vi "Text control 2 v6.7.vi"() -> ()   [LabVIEW 2016]
panel:
  in  "Tab Control":enum32{"Main", "Other parameters"}(tab)
  in  "Plot sample extrema vs time":bool
  out "Line running":i32
  out "Total lines":i32
  out "Path":path=path "C:/users/rlp38/09Apr2009LTtesting/test2.txt"
  out "I vs Vg":cluster{"Y data in":dbl[], "X data in":dbl[]}[](graph)
  out "Is max":dbl format="%.2e"
  out "Id max":dbl format="%.2e"
  out "Ig max":dbl format="%.2e"
  out "Imax vs time":cluster{"Y data in":dbl[], "X data in":dbl[]}[](graph)
  out "Imin vs time":cluster{"Y data in":dbl[], "X data in":dbl[]}[](graph)
  out "I vs Vd":cluster{"Y data in":dbl[], "X data in":dbl[]}[](graph)
  in  "Script":string="#pulsedstressV d 0.03 20 0 0.5 0.0827 5\n#\n#itime m\n#gaterangemode a\n#drainrangemode a\n#pulsed on 0.05 0 0.02\n#transfer d -10 40 1 5 40 35\n#transfer d -10 40 1 5 40 35\n#transfer d -10 40 1 5 40 35\n#output d 0 40 20 0 40 1\n#\n#\n#sample 1 0.008 221 6 0.003\n#samplei 400e-6 200 6 0.002 0.1\n#vsu2pulse -10 4\n#\n#stressV 0.016 0.03 2e-4 0.1e-3 11\n#stressI 220e-7 0.08 15\n#transfer s -1 1 0.5 -0.005 0.005 0.005\n#output s 0 0 0 -0.008 0.008 0.002"
  out "Command running:":string
  out "Serial port data":string
  out "Elapsed Time":dbl caption="Elapsed Time (s)"
  in  "Time Units":u16(ring)=1 items=["Seconds", "Minutes", "Hours"]
  in  "Time Offset":dbl caption="Set Start Time (s)"
  in  "Reset":bool
  in  "Auto Reset":bool
  in  "integration time":u32(slide) max=2 step=1 scale=0.0..2.0
  out "Is on":dbl format="%.2e"
  out "Id on":dbl format="%.2e"
  out "Ig on":dbl format="%.2e"
  out "Ion vs time":cluster{"Y data in":dbl[], "X data in":dbl[]}[](graph)
  out "Ioff vs time":cluster{"Y data in":dbl[], "X data in":dbl[]}[](graph)
  out "Ig min":dbl format="%.2e"
  out "Id min":dbl format="%.2e"
  out "Is min":dbl format="%.2e"
  out "Is off":dbl format="%.2e"
  out "Id off":dbl format="%.2e"
  out "Ig off":dbl format="%.2e"
  in  "Integration time (long)":dbl=0.32 min=0.04 max=2.0 step=0.02 format="%.2f"
  in  "Integration time (short)":dbl=0.0019 min=8e-05 max=0.0019 step=8e-05 format="%^.0e"
  in  "Drain: Compliance":dbl=0.001 format="%.8f"
  in  "Gate: Compliance":dbl=0.001 format="%.8f"
  in  "Interrupt scan":bool
  in  "Interrupt program":bool
  in  "Plot output curve extrema vs time":bool
  in  "Plot transfer curve extrema vs time":bool
  out "I vs time (Bias Stress)":cluster{"Y data in":dbl[], "X data in":dbl[]}[](graph)
  in  "Gate Range\nmode":u16(ring) items=["Auto", "Limited", "Fixed"]
  in  "Gate Range":u8(slide)=6 max=11 scale=0.0..11.0
  in  "Source/Drain\nRange mode":u16(ring) items=["Auto", "Limited", "Fixed"]
  in  "Source/Drain Range":u8(slide)=6 max=11 scale=0.0..11.0
  in  "Panel Controls":T1={"Emergency Stop"=refnum, "TransGraph Max"=1e-05, "Text/Graph (text=false)"=TRUE} {"TransGraph Max" format="%.2e"}
  in  "Panel Controls 2":T2={"Emergency Stop"=refnum, "TransGraph Max"=1e-05, "Text/Graph (text=false)"=TRUE, "TransGraph Min"=1e-11} {"TransGraph Min" format="%.2e"; "TransGraph Max" format="%.2e"}
  out "error out":errorcluster
  in  "Delay before read (ms)":u32=1000
  in  "byte count":u32=64
  in  "Serial End Mode for Reads":u16(ring)=2 items=["None", "LastBit", "TermChar"]
  in  "Timeout (ms)":u32=10000
  in  "Enable Termination\nChar (T)":bool=TRUE
  in  "Termination char\n(0xA = '\\n' = LF)\n(0xD = '\\r' = CR)":u8=13 format="%.0x"
  in  "flow control":u16(ring) items=["None"=0, "XON/XOFF"=1, "RTS/CTS"=2, "DTR/DSR"=4]
  in  "stop bits":u16(ring)=10 items=["1.0"=10, "1.5"=15, "2.0"=20]
  in  "parity":u16(ring) items=["None", "Odd", "Even", "Mark", "Space"]
  in  "data bits":u16=8 min=5 max=8 step=1
  in  "VISA resource name":refnum<visa-resource-name>="COM6"
  in  "baud rate":u32=9600
  out "Timings Indicator":T3
  in  "Timings (overwritten by the Front Panel)":T4={"integration time"=0, "Short/Long integration time"=0.00064, "hold time (sec)"=0.0, "delay time (sec)"=0.0, "Step Time (0 disables)"=0.0, "sweep method"=0, "Pulse period"=0.005, "Base voltage"=0.0, "Pulse width"=0.0005} {"Pulse width" min=0.0005 max=0.1 step=0.0001 format="%.4f"; "Base voltage" format="%^.4e"; "Pulse period" min=0.005 max=1.0 step=0.0001 format="%.4f"; "sweep method" items=["Continuous", "Pulsed"]; "Step Time (0 disables)" format="%.2f"; "delay time (sec)" format="%.4f"; "hold time (sec)" format="%.4f"; "Short/Long integration time" format="%^.0e"; "integration time" scale=0.0..2.0}
  in  "SMU4":cluster{"on/off":bool, "Voltage":dbl} {"Voltage" min=-100.0 max=100.0 format="%.2f"}
  in  "Full Reset":bool
  in  "Standby":T5
  out "SMU4 Indicator":cluster{"on/off":bool, "Voltage":dbl} {"Voltage" min=-100.0 max=100.0 format="%.2f"}
  in  "Gate":T6={"Gate Start"=0.0, "Gate Stop"=2.0, "Gate Step (linear only)"=1.0, "Gate Compliance"=0.0001, "Gate PComp"=0.0, "Range mode"=0, "Range"=6} {"Range" max=11 scale=0.0..11.0; "Range mode" items=["Auto", "Limited", "Fixed"]; "Gate PComp" format="%^.2e"; "Gate Compliance" format="%^.2e"; "Gate Step (linear only)" format="%^.4e"; "Gate Stop" format="%^.4e"; "Gate Start" format="%^.4e"}
  in  "Drain 2":T7={"Drain Start"=0.0, "Drain Stop"=2.0, "Drain Compliance"=0.0001, "Drain Step"=1.0, "Drain PComp"=0.0, "Range mode"=0, "Range"=6} {"Range" max=11 scale=0.0..11.0; "Range mode" items=["Auto", "Limited", "Fixed"]; "Drain PComp" format="%^.2e"; "Drain Step" format="%^.4e"; "Drain Compliance" format="%^.2e"; "Drain Stop" format="%^.4e"; "Drain Start" format="%^.4e"}
  # "Time"
  # "Syntax:\nitime [s|m|l] time(sec): [s|m|l] determines the integration time setting (small|medium|long) and time sets the value.\nNOTE: The value of the integration time has to be within the range allowed by its category (s|m|l), otherwise, the closest value will be used. (e.g. if the category is set to short but the time value is very long, the actual value used will be the maximum short integration time.\nIntegration times:\n    Short: Default: 640 us. Range: 8E-5 - 1.92E-3 seconds.\n    Medium: Fixed at 1 NPL cycle (0.02 seconds).\n    Long: Default: 16 NPL cycles (0.32 seconds). Range: 2-100 NPL cycles (0.04 seconds - 2 seconds).\ngaterangemode [a|l|f]\ndrainrangemode [a|l|f]\npulsed [on|off] PulsePeriod(sec) PulseBaseVoltage PulseONWidth(sec)\nstandby [on l off]\nwait NumMilliseconds\nwait-min NumMinutes\n# texthere = comment\nSMU4 [ON|OFF] Voltage\ntransfer [s|d] VgStart VgStop VgStep VdStart VdStop VdStep\noutput [s|d] VgStart VgStop VgStep VdStart VdStop VdStep\nsample Vg Vd NumSamples Time(s) SampleInterval(s)\nsamplei Idg NumSamples Time(s) SampleInterval(s) VDGcompliance\n100 samples is approximately 13 seconds with medium integration\n# if in doubt use SampleInterval(s) = 0.004\n    NOTE: When doing bias stress measurements, set the Time Units to \"Seconds\", as the \"sample\" command has been configured to give the output to seconds.\nstressV VG VD IGcompliance IDcompliance Duration(sec)\nstressI IDG VDGcompliance Duration(sec)\nvsu2pulse Bias Duration(s)\npulsedstressV [s|d] VEstop VgON VgOFF Period(s) PulseONwidth(s) Vd\nsample-fpp Vg Vd NumSamples Time\nresample-fpp Vg Vd\ntransfer-fpp [s|d] VgStart VgStop VgStep VdStart VdStop VdStep\noutput-fpp [s|d] VgStart VgStop VgStep VdStart VdStop VdStep\nserial SerialPortCommand"
  # "1\n2\n3\n4\n5\n6\n7\n8\n9\n10\n11\n12\n13\n14\n15\n16\n17\n18\n19\n20"
  # "Serial port settings"
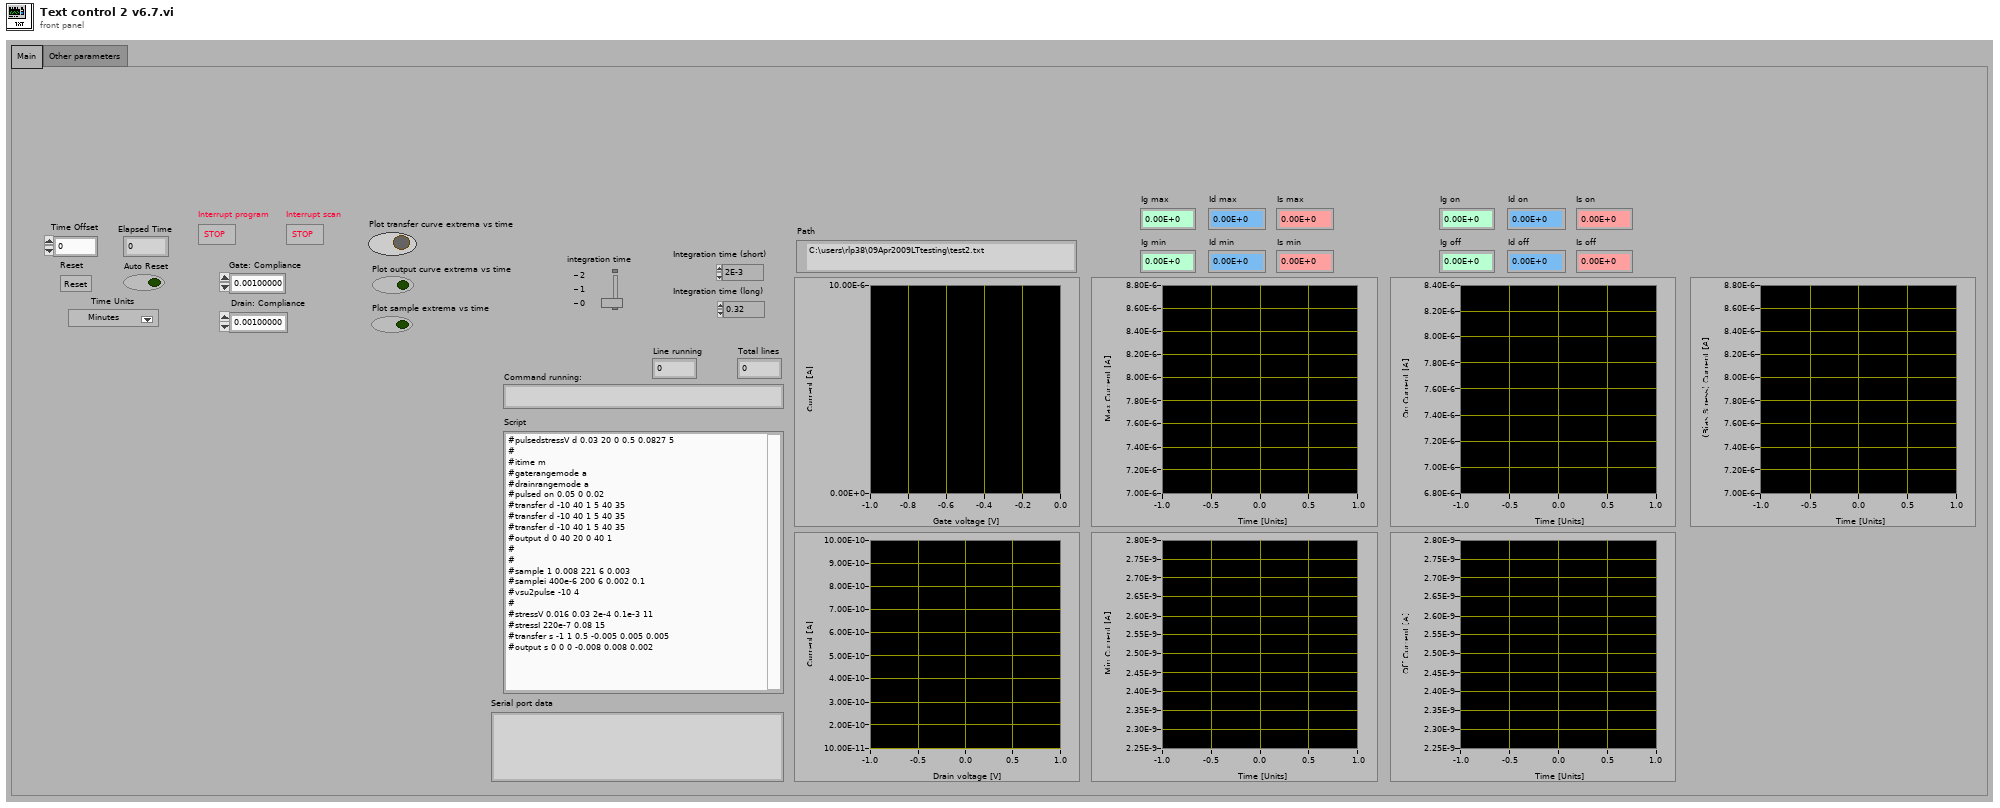
[diagram p1: front panel]
types:
  T1 = cluster{"Emergency Stop":refnum<vi>, "TransGraph Max":dbl, "Text/Graph (text=false)":bool}
  T2 = cluster{"Emergency Stop":refnum<vi>, "TransGraph Max":dbl, "Text/Graph (text=false)":bool, "TransGraph Min":dbl}
  T3 = cluster{"integration time (0:s, 1:m, 2:l)":u32, "Short/Long integration time":dbl, "hold time (sec)":dbl, "delay time (sec)":dbl, "Step Time (0 disables)":dbl, "sweep method":u16, "Pulse period":dbl, "Base voltage":dbl, "Pulse width":dbl}
  T4 = cluster{"integration time":u32, "Short/Long integration time":dbl, "hold time (sec)":dbl, "delay time (sec)":dbl, "Step Time (0 disables)":dbl, "sweep method":u16, "Pulse period":dbl, "Base voltage":dbl, "Pulse width":dbl}
  T5 = cluster{"Gate Standby":bool, "Drain Standby":bool}
  T6 = cluster{"Gate Start":dbl, "Gate Stop":dbl, "Gate Step (linear only)":dbl, "Gate Compliance":dbl, "Gate PComp":dbl, "Range mode":u16, "Range":u8}
  T7 = cluster{"Drain Start":dbl, "Drain Stop":dbl, "Drain Compliance":dbl, "Drain Step":dbl, "Drain PComp":dbl, "Range mode":u16, "Range":u8}
  T8 = enum16{"open", "replace", "create", "open or create", "replace or create", "replace or create with confirmation"}
  T9 = cluster{"V2 Start":dbl, "V2 Step":dbl, "Number of points":i32}
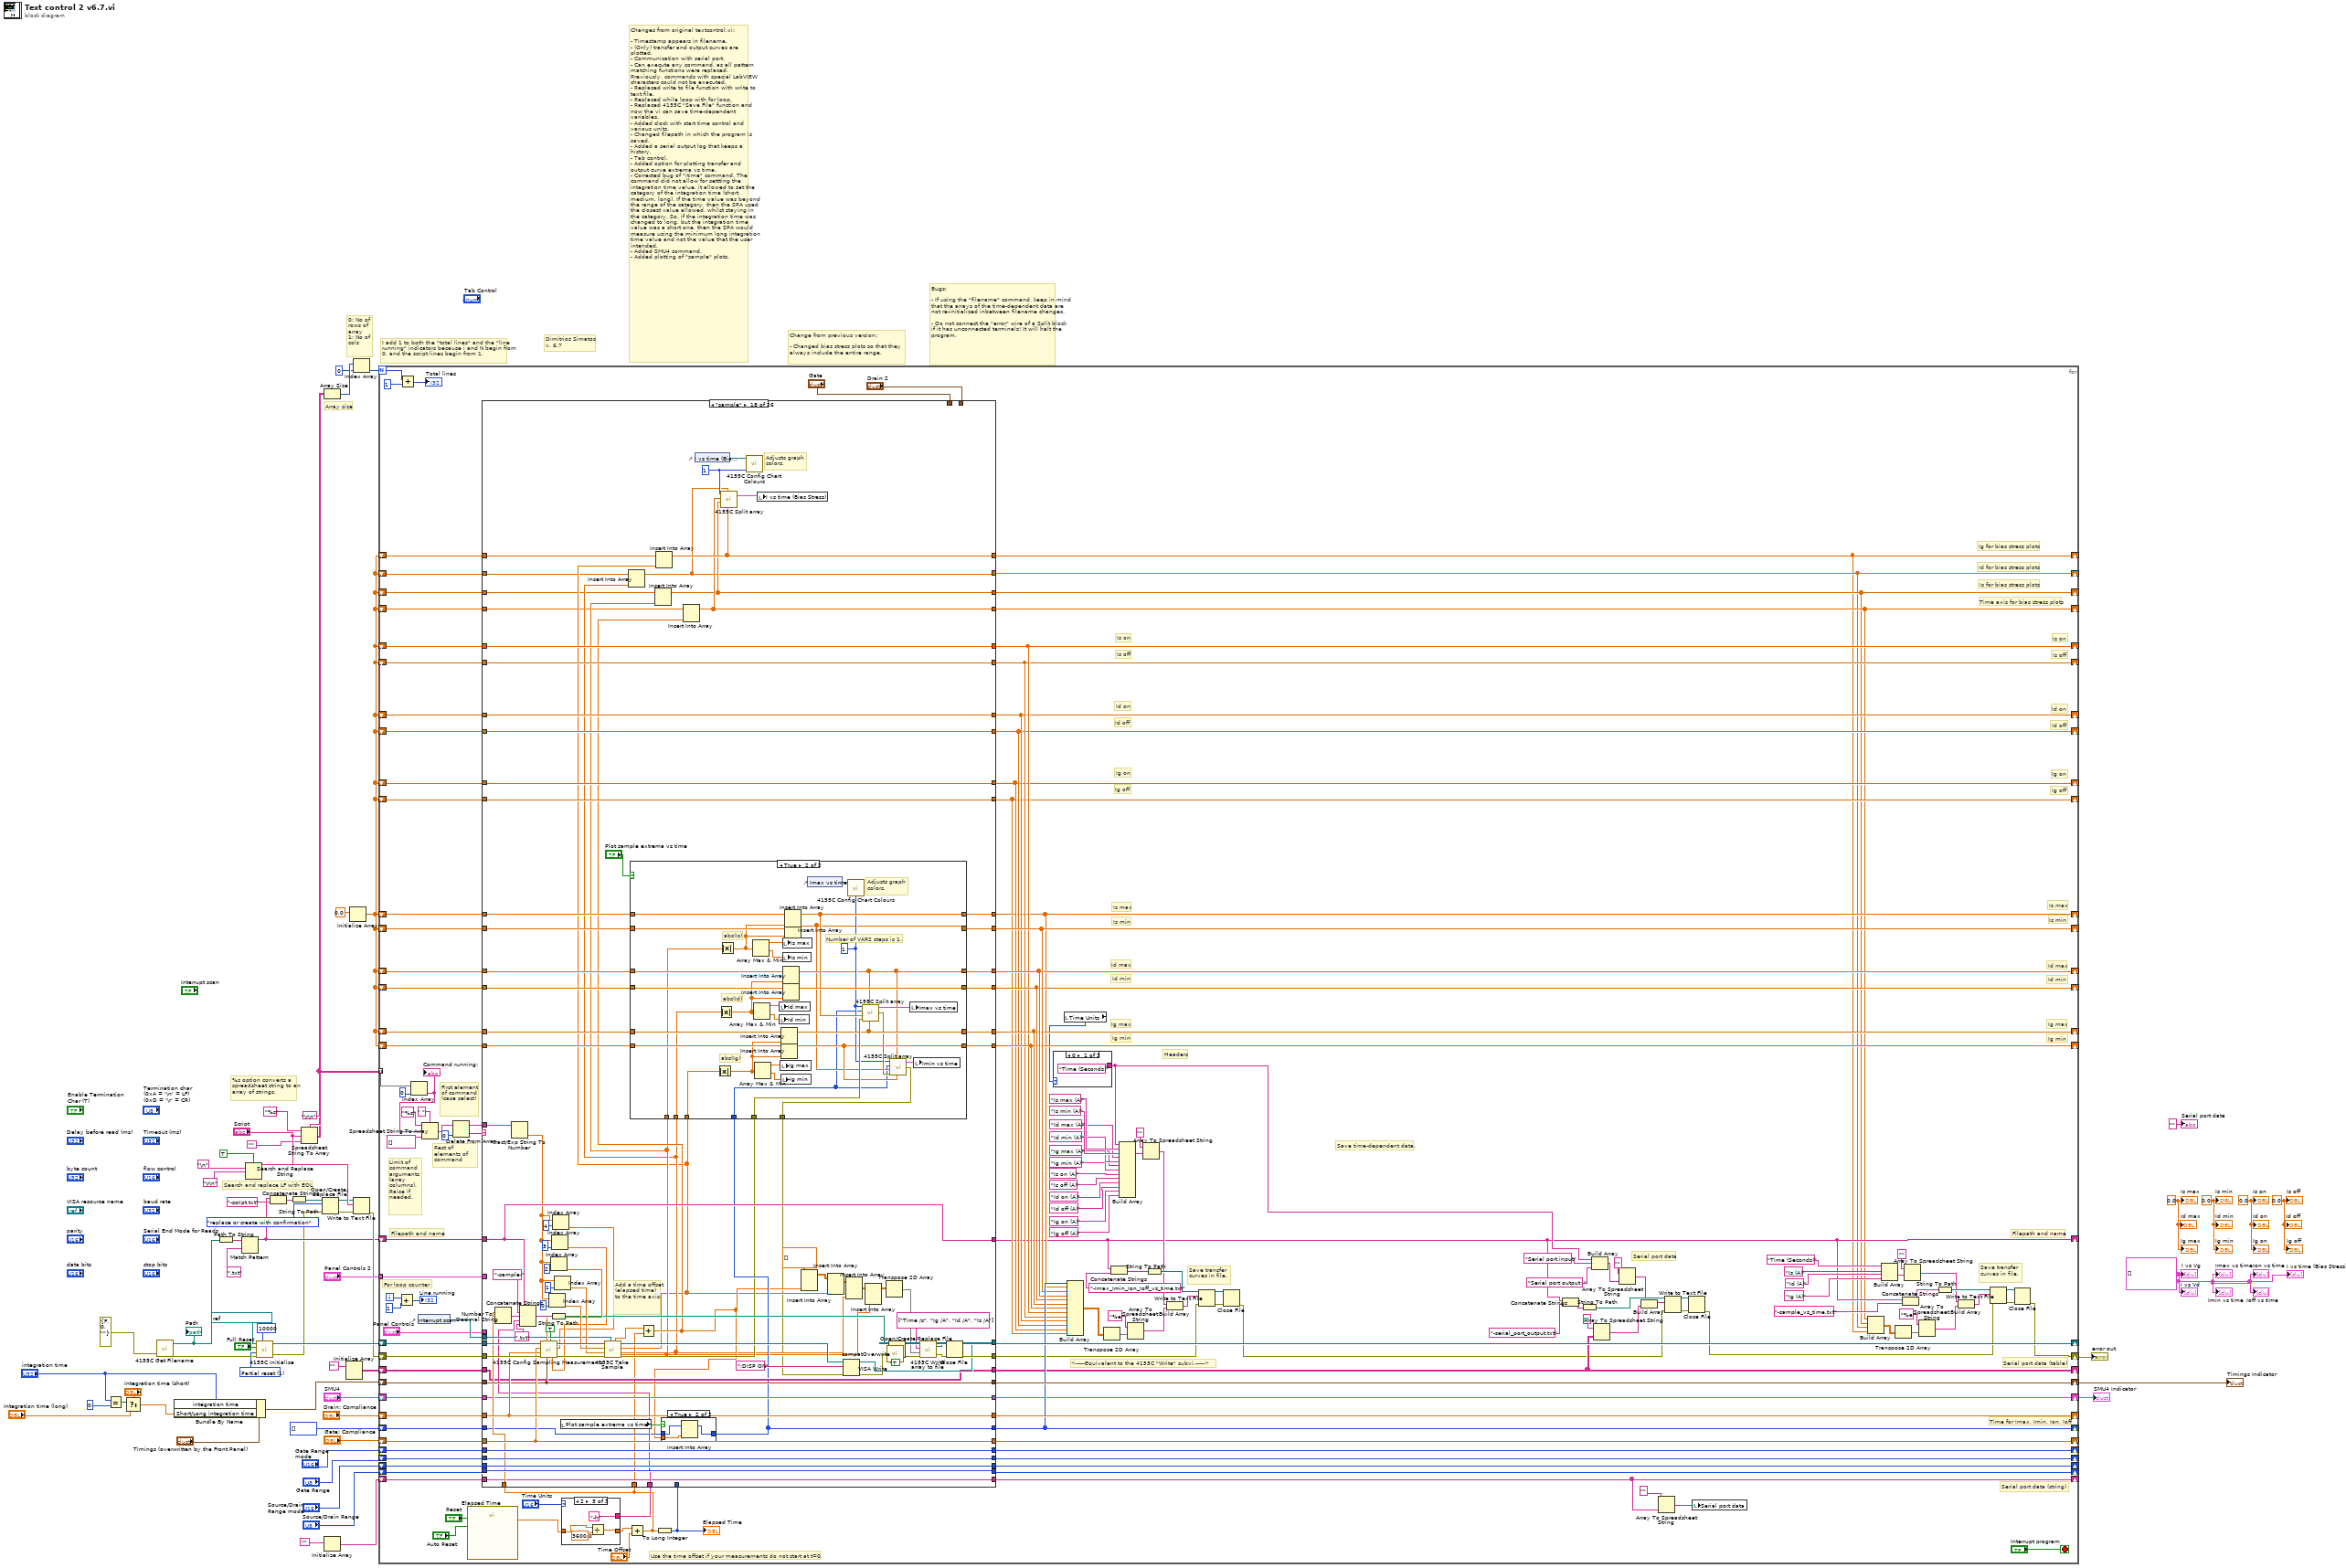
[diagram p0: block diagram]
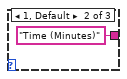
[diagram p2: hidden frame]
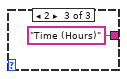
[diagram p3: hidden frame]
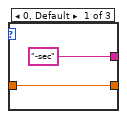
[diagram p4: hidden frame]
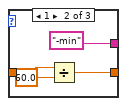
[diagram p5: hidden frame]
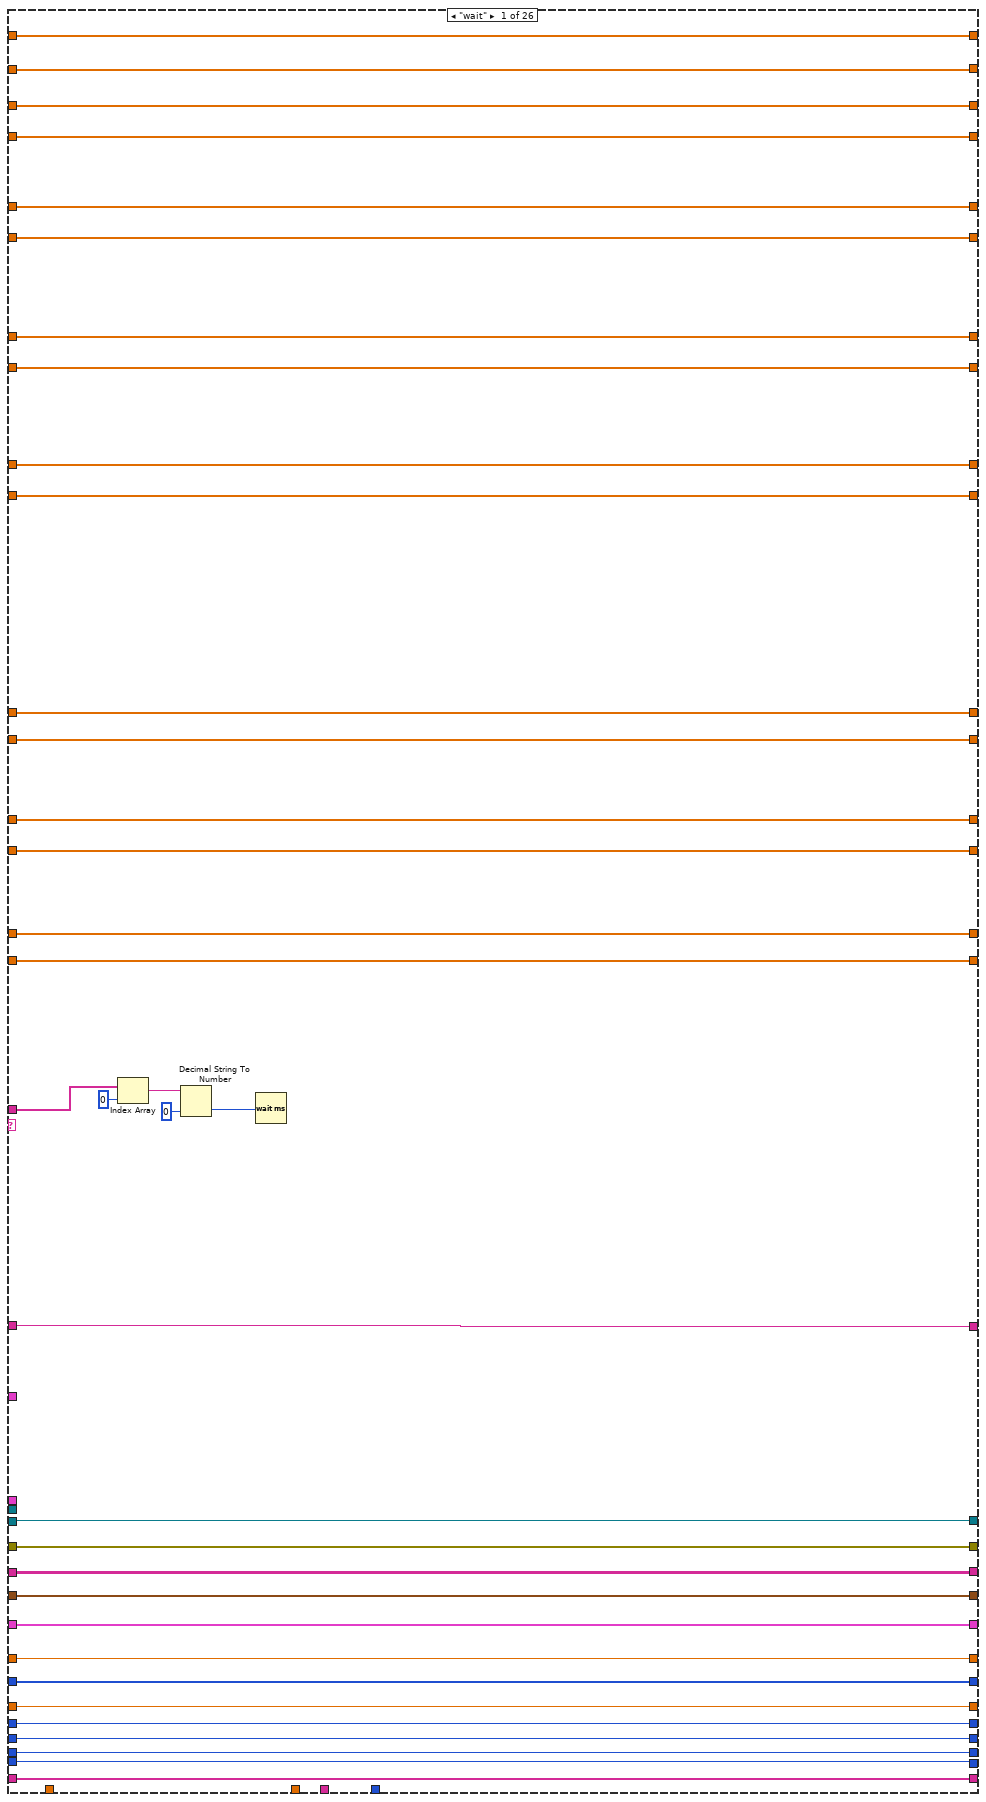
[diagram p6: hidden frame]
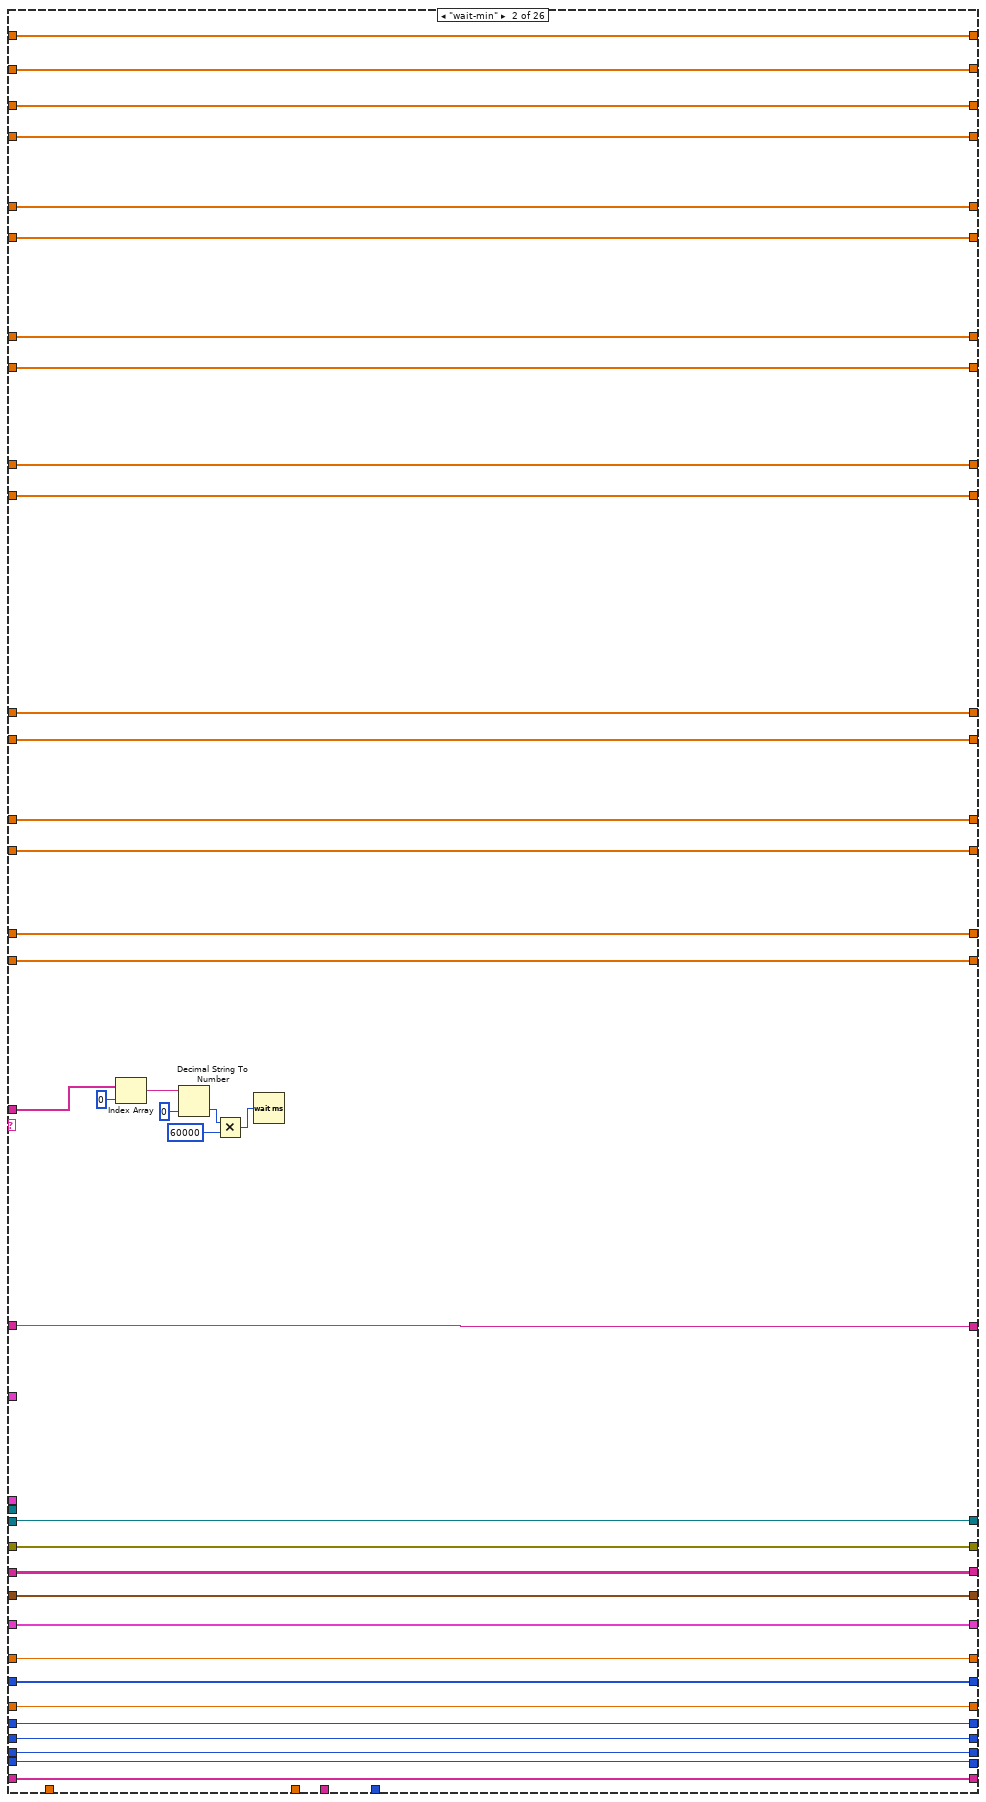
[diagram p7: hidden frame]
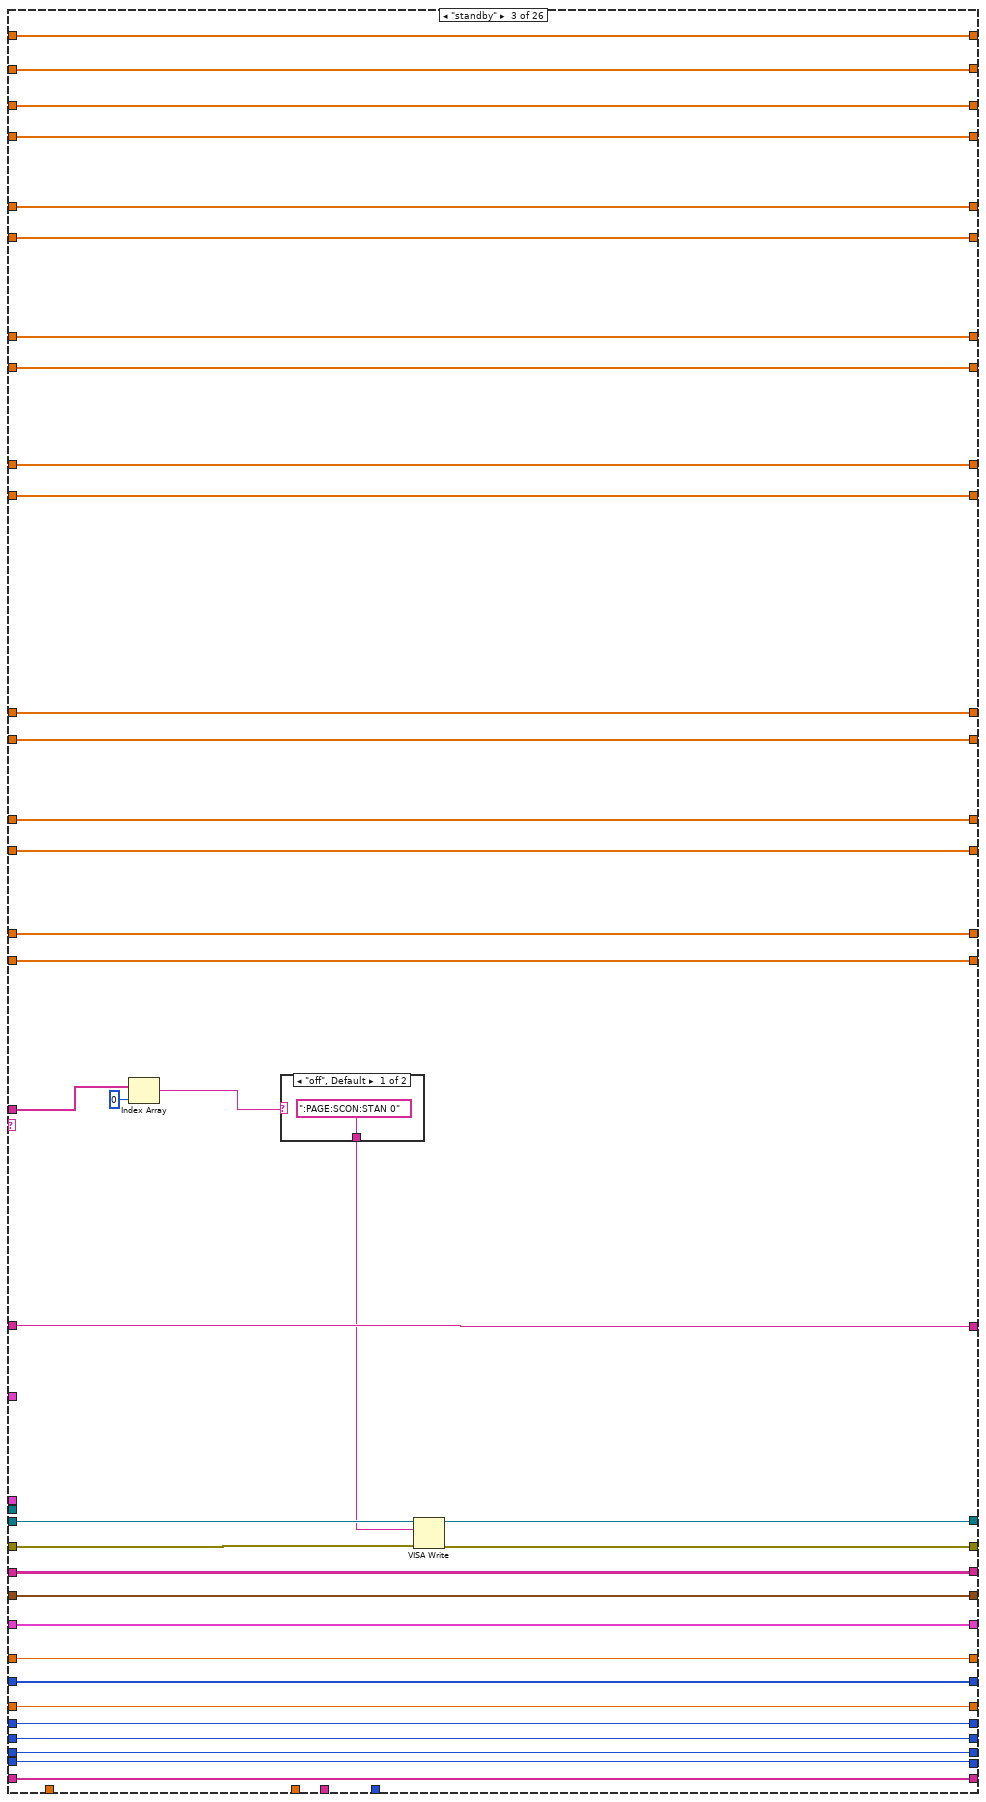
[diagram p8: hidden frame]
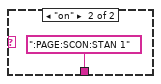
[diagram p9: hidden frame]
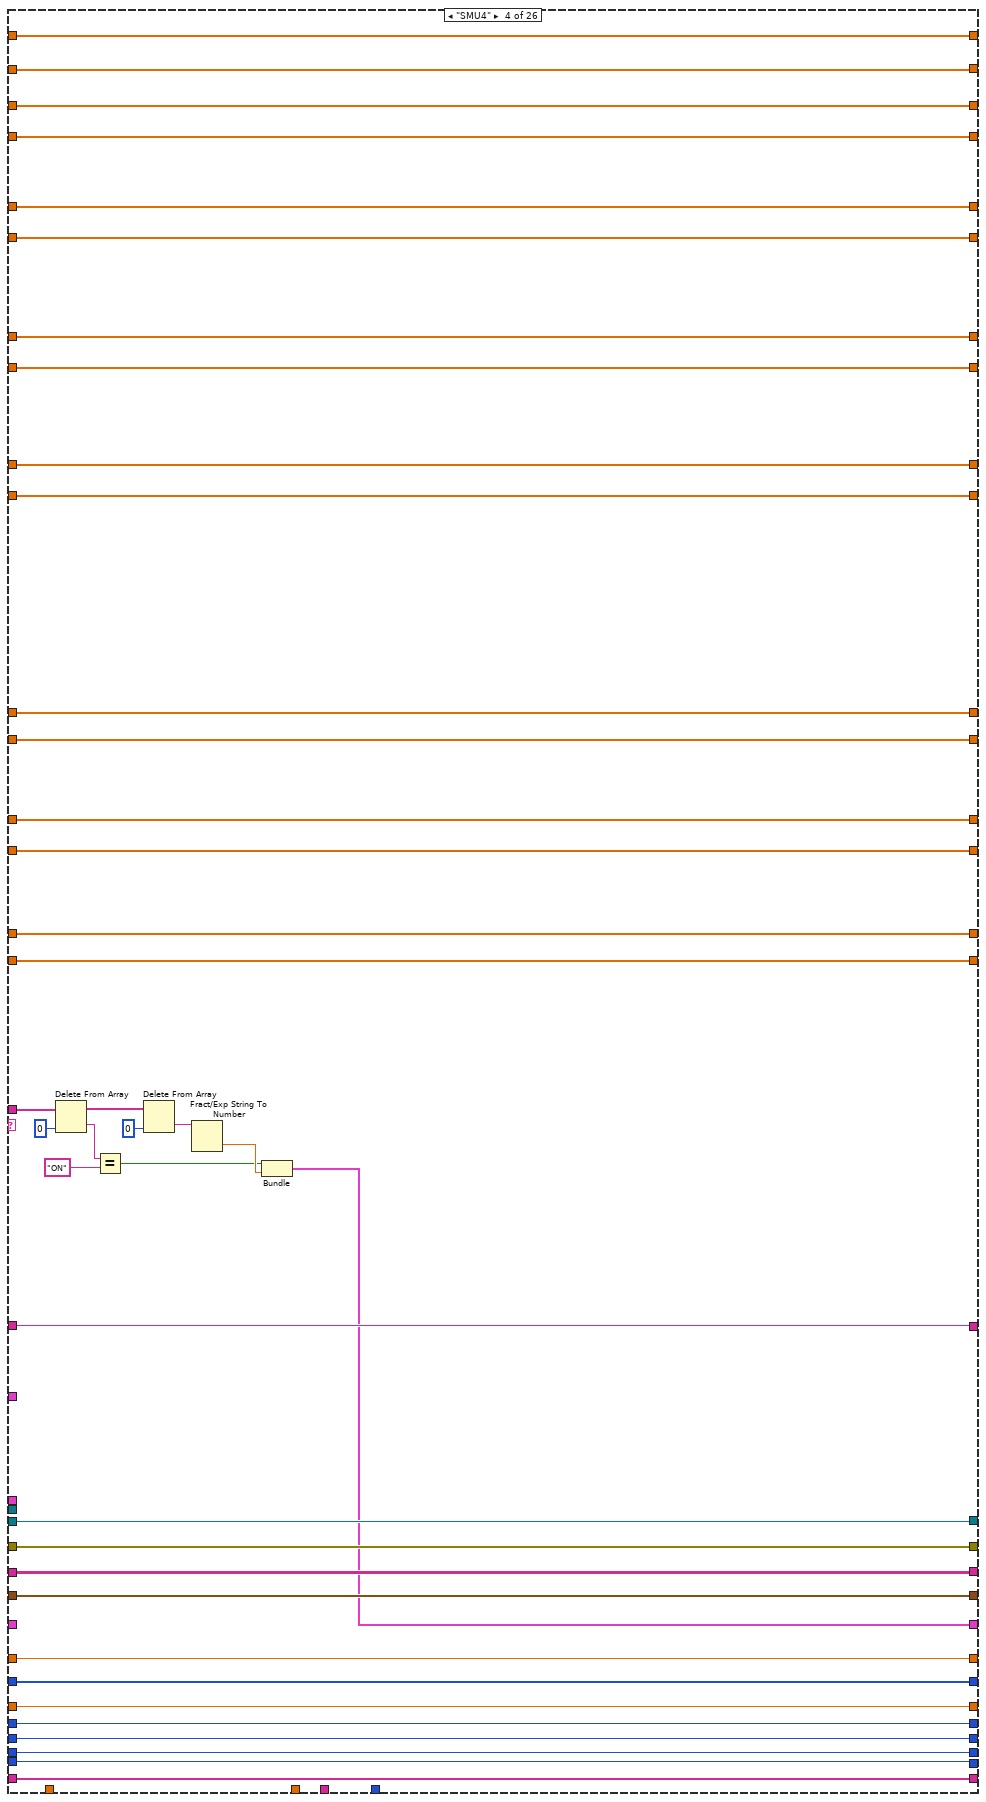
[diagram p10: hidden frame]
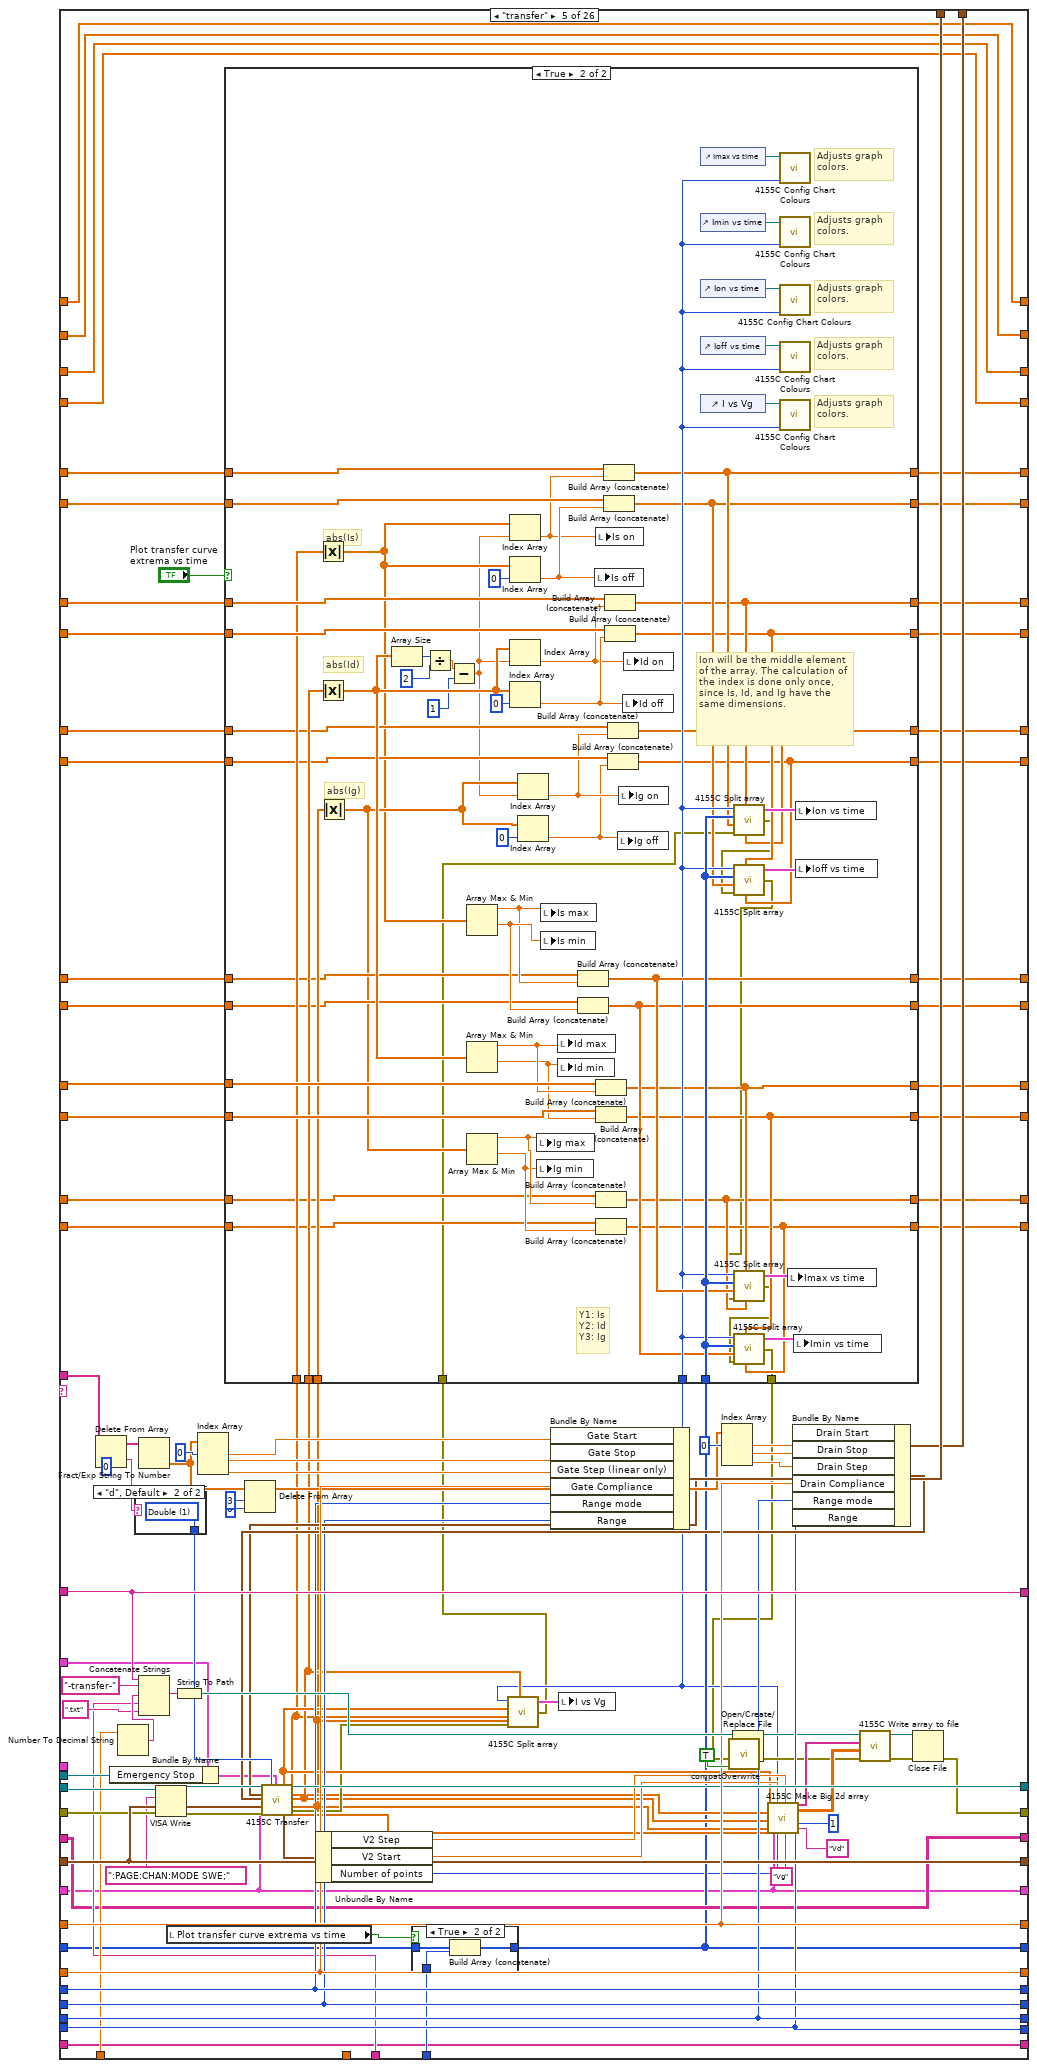
[diagram p11: hidden frame]
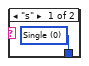
[diagram p14: hidden frame]
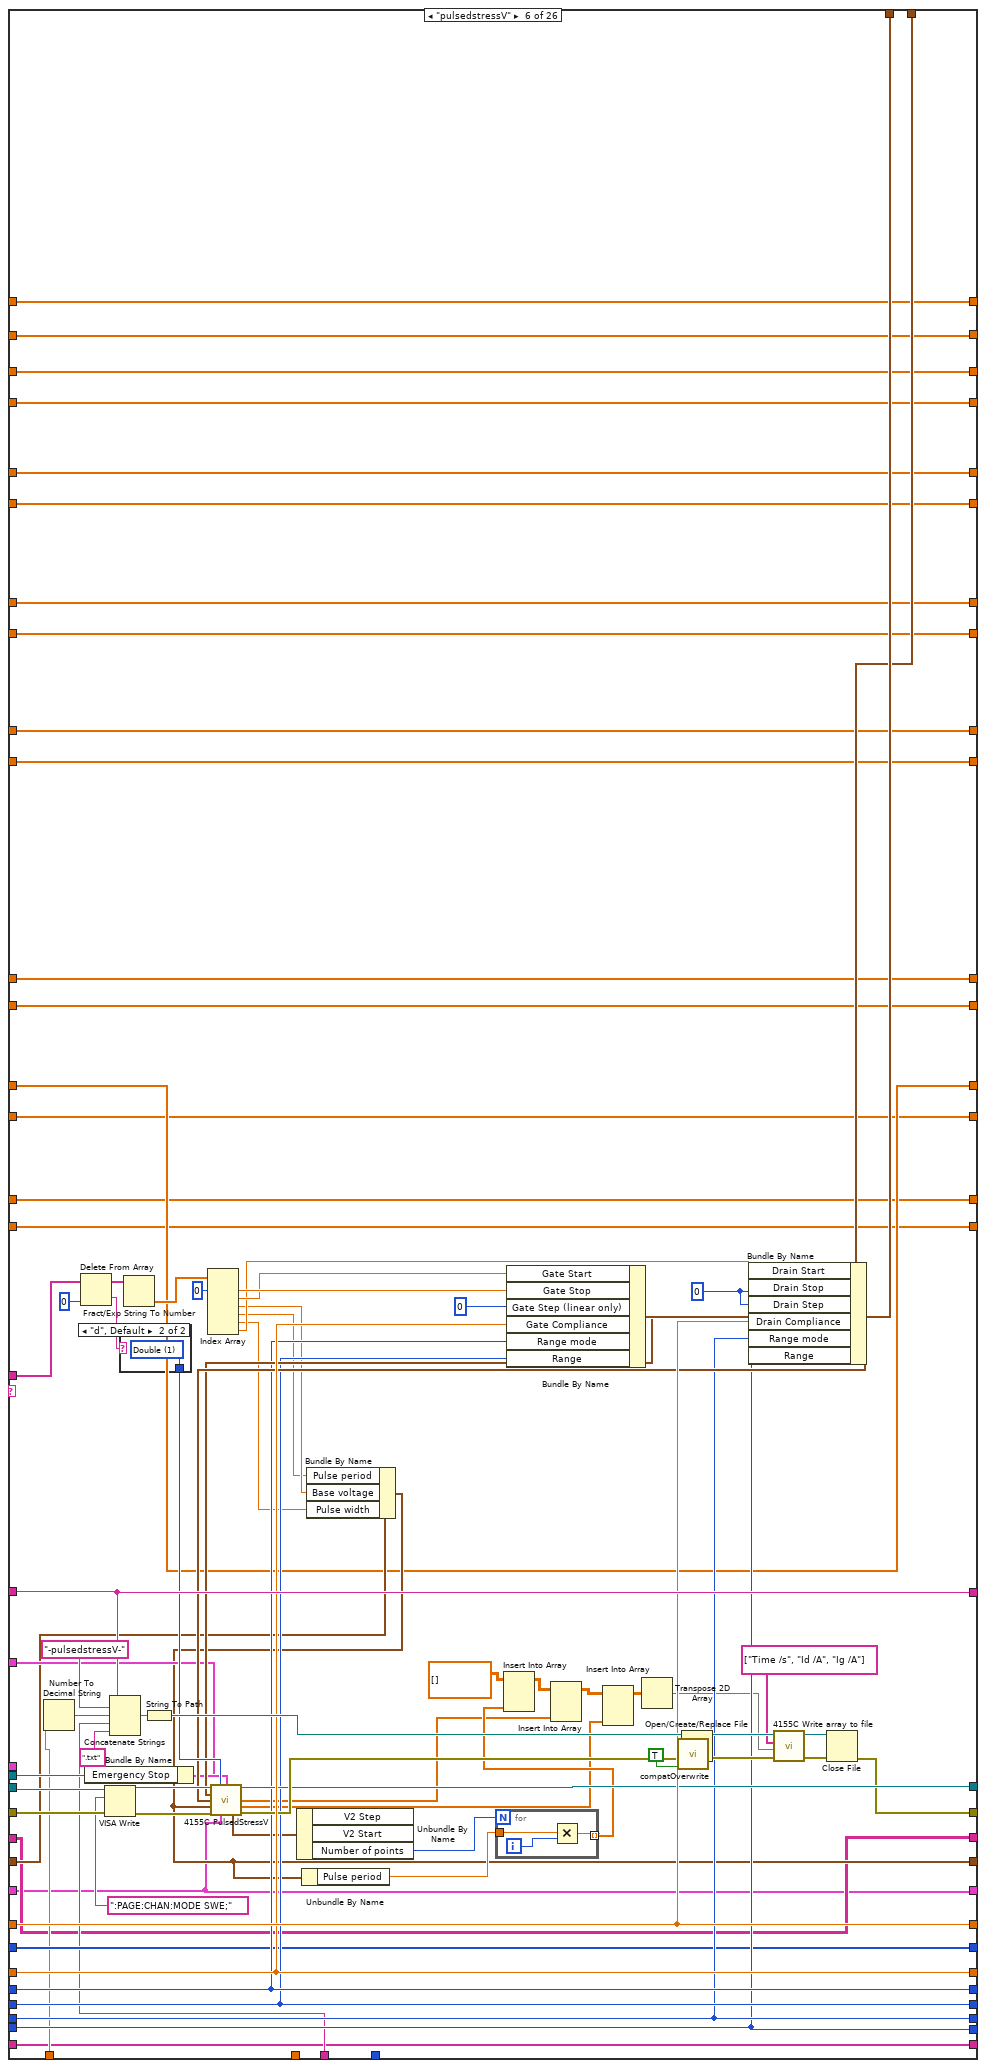
[diagram p15: hidden frame]
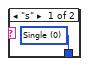
[diagram p16: hidden frame]
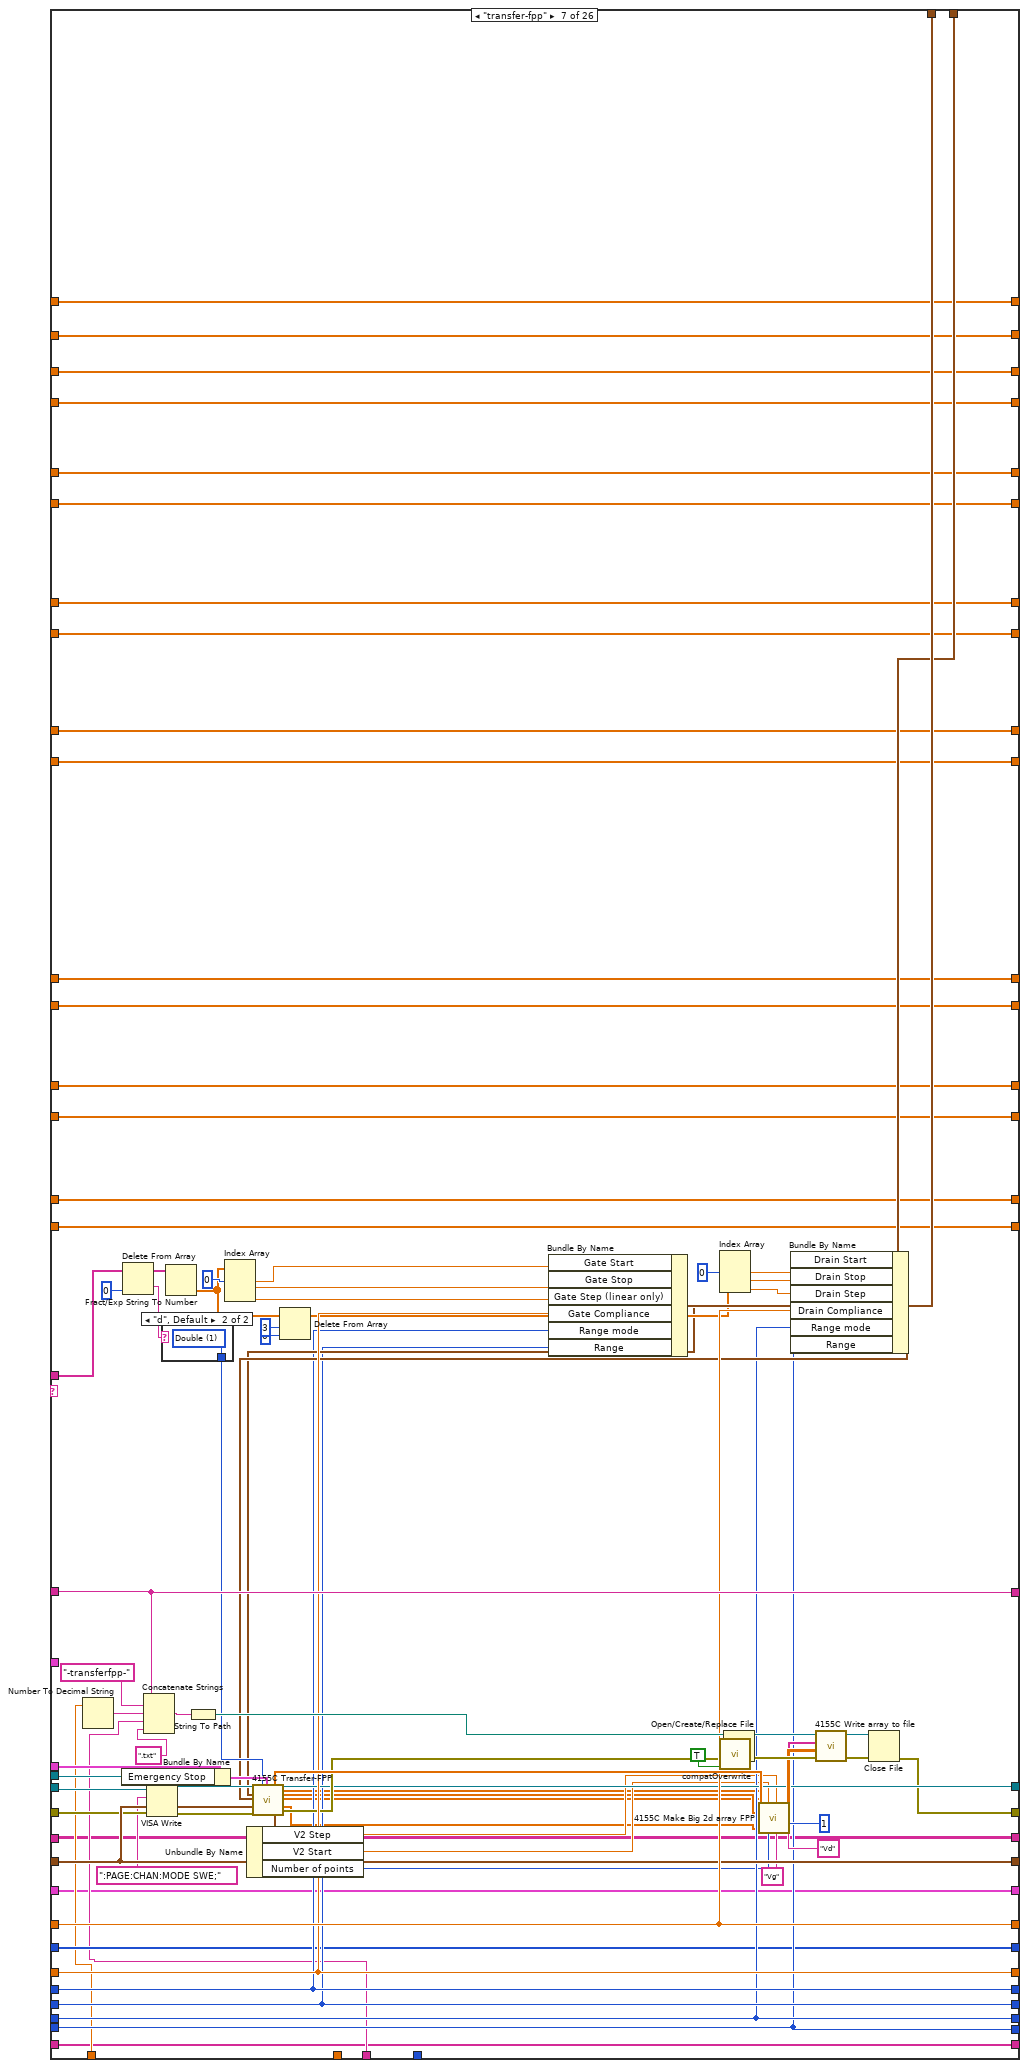
[diagram p17: hidden frame]
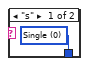
[diagram p18: hidden frame]
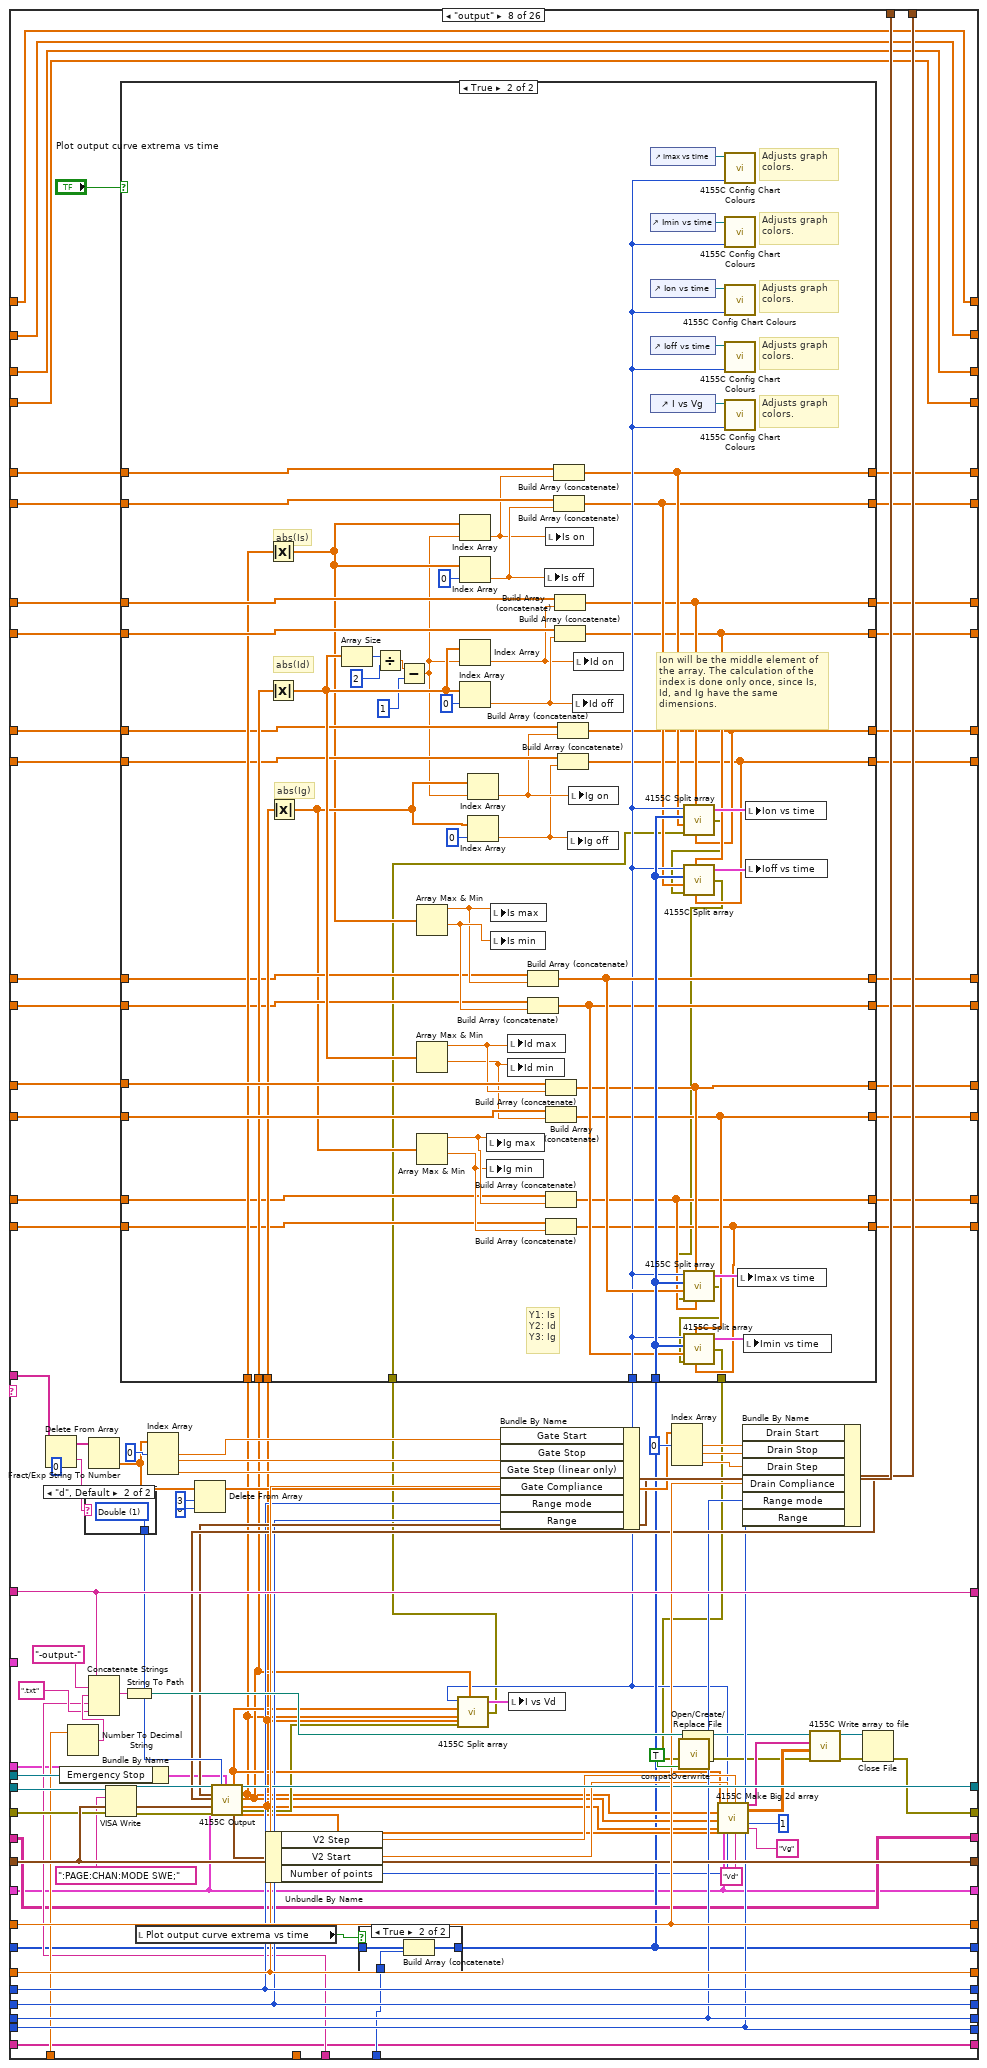
[diagram p19: hidden frame]
diagram:
  w2 = cluster{"Y data in":dbl[], "X data in":dbl[]}[] [] ("I vs Vg")
  w10 = 0.0 ("Is off")
  w11 = 0.0 ("Is on")
  w12 = 0.0 ("Is min")
  w13 = 0.0 ("Is max")
  w58 = u16 1 items=["Reset All", "Partial reset"] ("Type of reset")
  # "Change from previous version:\n\n- Changed bias stress plots so that they always include the entire range."
  # "I add 1 to both the \"total lines\" and the \"line running\" indicators because i and N begin from 0, and the script lines begin from 1."
  # "Bugs:\n\n- If using the \"filename\" command, keep in mind that the arrays of the time-dependent data are not re-initialized inbetween filename changes. \n\n- Do not connect the \"error\" wire of a Split block if it has unconnected terminals! It will halt the program."
  # "Array size"
  # "%s option converts a spreadsheet string to an array of strings."
  # "0: No of rows of array\n1: No of cols"
  # "Dimitrios Simatos\nv. 6.7"
  # "Changes from original textcontrol.vi:\n\n- Timestamp appears in filename.\n- (Only) transfer and output curves are plotted.\n- Communication with serial port.\n- Can execute any command, as all pattern matching functions were replaced. Previously, commands with special LabVIEW characters could not be executed.\n- Replaced write to file function with write to text file.\n- Replaced while loop with for loop.\n- Replaced 4155C \"Save File\" function and now the vi can save time-dependent variables.\n- Added clock with start time control and various units.\n- Changed filepath in which the program is saved.\n- Added a serial output log that keeps a history.\n- Tab control.\n- Added option for plotting transfer and output curve extrema vs time.\n- Corrected bug of \"itime\" command. The command did not allow for settting the integration time value, it allowed to set the category of the integration time (short, medium, long). If the time value was beyond the range of the category, then the SPA used the closest value allowed, whilst staying in the category. So, if the integration time was changed to long, but the integration time value was a short one, then the SPA would measure using the minimum long integration time value and not the value that the user intended.\n- Added SMU4 command.\n- Added plotting of \"sample\" plots."
  # "Search and replace LF with EOL"
  n1 = Equal?(x="integration time", y=u32 0) -> (x = y?=w59:bool)
  n2 = Select(t="Integration time (short)", s=w59, f="Integration time (long)") -> (s? t:f=w18:dbl)
  n3 = call "4155C Get Filename.vi"("error in (no error)"=errorcluster {"status"=FALSE, "code"=0, "source"=""}) -> ("error out"=w53:errorcluster, "path"=w28:path)  [unwired: 2 in, 1 out]
  "Path" <- w28
  n4 = Bundle By Name(cluster="Timings (overwritten by the Front Panel)", "integration time"="integration time", "Short/Long integration time"=w18) -> (w51:T4)
  n5 = Path To String(path=w28) -> (string=w29:string)
  n6 = Match Pattern(string=w29, regular expression=".txt") -> (before substring=w16:string)  [unwired: 1 in, 3 out]
  n7 = Search and Replace String(replace all?=TRUE ("replace all? (F)"), input string="Script", search string="\n", replace string="\r\n") -> (result string=w41:string)  [unwired: 4 in, 3 out]
  n8 = call "4155C Initialise.vi"("VISA resource name in"=refnum<visa-resource-name> "GPIB0::14::INSTR", "Reset"="Full Reset", "Type of reset"=w58, "error in (no error)"=w53, "VISA Timeout Value"=u32 10000) -> ("VISA Resource Name out"=w52:refnum<visa-resource-name>, "error out"=w8:errorcluster)
  n9 = Concatenate Strings(w16, "-script.txt" ("string")) -> (w17:string)
  n10 = String To Path(string=w17) -> (path=w6:path)
  n11 = Spreadsheet String To Array(delimiter (Tab)="\r\n", format string="%s", spreadsheet string="Script", array type (2D Dbl)="") -> (array=w32:string[][])
  n12 = Open/Create/Replace File(file path (use dialog)=w6, error in=w8, operation (0:open)=T8."replace or create with confirmation") -> (refnum out=w5:refnum<file>, error out=w7:errorcluster)  [unwired: 3 in, 1 out]
  n13 = Array Size(array=w32) -> (size(s)=w36:i32[])
  n14 = Initialize Array("") -> (w22:string[])  [unwired: 1 in]
  n15 = Initialize Array("") -> (w20:string[][])  [unwired: 2 in]
  n16 = Initialize Array(0.0 ("element")) -> (w1:dbl[])  [unwired: 1 in]
  n17 = Index Array(array=w36, index=0) -> (element=w34:i32)
  n18 = Write to Text File(file (use dialog)=w5, text=w41, error in=w7) -> (error out=w25:errorcluster)  [unwired: 1 in, 2 out]
  n19 = for {
    N: w34 -> [w159]
    shift-left: "Source/Drain Range" -> [w199]
    shift-right: [w195] -> _
    shift-left: "Source/Drain\nRange mode" -> [w200]
    shift-right: [w196] -> _
    shift-left: "Gate Range" -> [w201]
    shift-right: [w197] -> _
    shift-left: "Gate Range\nmode" -> [w202]
    shift-right: [w198] -> _
    shift-left: "Gate: Compliance" -> [w211]
    shift-right: [w207] -> _
    shift-left: "Drain: Compliance" -> [w212]
    shift-right: [w208] -> _
    shift-left: w51 -> [w213]
    shift-right: [w209] -> w19
    shift-left: w25 -> [w214]
    shift-right: [w69] -> w27
    shift-left: w52 -> [w215]
    shift-right: [w210] -> _
    shift-left: w16 -> [w216]
    shift-right: [w68] -> _
    tunnel: "Panel Controls 2" -> [w193]
    shift-right: [w111] -> _
    shift-left: w1 -> [w192]
    shift-right: [w146] -> _
    shift-left: i32[] [] -> [w188]
    tunnel: w32 -> [w187] mode=indexing
    shift-right: [w110] -> _
    shift-left: w1 -> [w164]
    shift-right: [w141] -> _
    shift-left: w22 -> [w151]
    shift-right: [w142] -> _
    shift-left: w20 -> [w144]
    shift-right: [w104] -> _
    shift-left: w1 -> [w132]
    shift-right: [w105] -> _
    shift-left: w1 -> [w131]
    shift-right: [w109] -> _
    shift-left: w1 -> [w120]
    shift-right: [w108] -> _
    shift-left: w1 -> [w119]
    shift-right: [w102] -> _
    shift-left: w1 -> [w118]
    shift-right: [w112] -> _
    shift-left: w1 -> [w117]
    shift-right: [w103] -> _
    shift-left: w1 -> [w116]
    shift-right: [w101] -> _
    shift-left: w1 -> [w115]
    shift-right: [w107] -> _
    shift-left: w1 -> [w114]
    shift-right: [w106] -> _
    shift-left: w1 -> [w113]
    shift-right: [w94] -> w3
    shift-left: "SMU4" -> [w194]
    shift-right: [w64] -> _
    shift-left: w1 -> [w91]
    shift-right: [w65] -> _
    shift-left: w1 -> [w90]
    shift-right: [w66] -> _
    shift-left: w1 -> [w89]
    shift-right: [w67] -> _
    shift-left: w1 -> [w88]
    i -> [w154]
    stop <- "Interrupt program" stop-if-true
    # "Ig for bias stress plots"
    # "Id for bias stress plots"
    # "Is for bias stress plots"
    # "Time axis for bias stress plots"
    # "Save transfer curves in file."
    # "Is off"
    # "Is on"
    # "Ig off"
    # "Ig on"
    # "Is min"
    # "Is max"
    # "Ig min"
    # "Ig max"
    # "Id min"
    # "Id max"
    # "Id off"
    # "Id on"
    # "Is off"
    # "Is on"
    # "Ig off"
    # "Ig on"
    # "Is min"
    # "Is max"
    # "Ig min"
    # "Ig max"
    # "Id min"
    # "Id max"
    # "Id off"
    # "Id on"
    # "Filepath and name"
    # "Limit of command arguments (array columns). Raise if needed."
    # "Serial port data (string)"
    # "Serial port data (table)"
    # "Serial port data"
    # "For loop counter"
    # "<-----Equivalent to the 4155C \"Write\" subvi.----->"
    # "Headers"
    # "Save transfer curves in file."
    # "Filepath and name"
    # "Save time-dependent data."
    # "Use the time offset if your measurements do not start at t=0."
    # "Time for Imax, Imin, Ion, Ioff"
    # "Rest of elements of command"
    # "First element of command\n(case select)"
    n20 = Add(x=w154, y=1) -> (x+y=→"Line running":i32)
    n21 = Add(x=w159, y=1) -> (x+y=→"Total lines":i32)
    n22 = Index Array(array=w187, index=0 ("line index")) -> (element=w182:string)
    "Command running:" <- w182
    n23 = control-ref of="Interrupt scan"() -> (w206:refnum<vi>)
    n24 = Spreadsheet String To Array(delimiter (Tab)=" ", format string="%s", spreadsheet string=w182, array type (2D Dbl)=string[] []) -> (array=w180:string[])
    n25 = Delete From Array(array=w180, index=0) -> (deleted portion=w133:string, array with subset deleted=w179:string[])  [unwired: 1 in]
    n26 = call "Elapsed Time"("Reset"="Reset", "Auto Reset"="Auto Reset") -> ("Elapsed Time (s)"=w189:dbl)  [unwired: 10 in, 7 out]
    n27 = case shown="2" "Time Units" {
      tunnel: ["-sec" "-min" "-h"] -> w190
      tunnel: [w220 w224 w227] -> w160
      tunnel: w189 -> [w220 w223 w228]
      frame 0, Default {
      }
      frame 1 {
        n28 = Divide(x=w223, y=60.0) -> (x/y=w224:dbl)
      }
      frame 2 {
        n29 = Divide(x=w228, y=3600.0) -> (x/y=w227:dbl)
      }
    }
    n30 = Add(x=w160, y="Time Offset") -> (x+y=w92:dbl)
    n31 = To Long Integer(number=w92) -> (32bit integer=w93:i32)
    "Elapsed Time" <- w93
    n32 = case shown="\"sample\"" w133 {
      tunnel: w179 -> [w264 w301 w337 w353 w474 w585 w724 w843 w1003 w1035 w1108 w1153 w1196 w1235 w1267 _ _ w1446 w1566 _ w1667 w1729 w1789 w1877 w1957 w1995]
      tunnel: w216 -> [w259 w297 w335 w366 w481 w644 w732 w850 w1011 w1052 w1097 w1145 w1189 w1229 w1260 w1297 w1357 w1427 w1548 w1597 w1654 w1716 w1777 w1871 w1953 w1997]
      tunnel: w215 -> [w258 w296 w326 w365 w452 w629 w701 w821 w979 w1053 w1098 w1146 w1190 w1230 w1261 w1302 w1359 w1452 w1572 w1601 w1673 w1735 w1795 w1883 w1911 w2001]
      tunnel: w214 -> [w257 w295 w325 w364 w451 w628 w700 w820 w976 w1054 w1099 w1147 w1191 w1231 w1262 w1301 w1330 w1451 w1571 w1600 w1672 w1734 w1794 w1882 w1910 w2000]
      tunnel: w213 -> [w256 w294 w334 w362 w477 w605 w728 w846 w1007 w1062 w1107 w1144 w1188 w1228 w1259 w1300 w1354 w1419 w1540 w1606 w1647 w1709 w1770 w1870 w1952 w2002]
      tunnel: w212 -> [w255 w293 w333 w361 w479 w642 w730 w848 w1009 w1061 w1106 w1152 w1195 w1234 w1266 w1299 w1339 w1450 w1570 w1609 w1671 w1733 w1793 w1881 w1961 w2003]
      tunnel: w211 -> [w254 w292 w332 w359 w478 w641 w729 w847 w1008 w1060 w1105 w1151 w1194 w1233 w1265 w1298 w1340 w1428 w1549 w1608 w1655 w1717 w1778 w1872 w1954 w2005]
      tunnel: [w258 w296 w324 w365 w476 w639 w726 w845 w1005 w1053 w1098 w1146 w1190 w1230 w1261 w1302 w1359 w1420 w1522 w1599 w1648 w1710 w1771 w1823 w1913 w2001] -> w210
      tunnel: [w257 w295 w323 w364 w475 w638 w725 w844 w1004 w1054 w1099 w1147 w1191 w1231 w1262 w1301 w1329 w1429 w1523 w1598 w1656 w1718 w1779 w1822 w1912 w1999] -> w145
      tunnel: [w256 w294 w334 w362 w477 w601 w728 w846 w1007 w1055 w1100 w1144 w1188 w1228 w1259 w1300 w1354 w1419 w1540 w1606 w1647 w1709 w1770 w1870 w1952 w2002] -> w209
      tunnel: [w255 w293 w333 w361 w479 w642 w730 w848 w1009 w1061 w1106 w1152 w1195 w1234 w1266 w1299 w1339 w1450 w1570 w1609 w1671 w1733 w1793 w1881 w1961 w2003] -> w208
      tunnel: [w254 w292 w332 w359 w478 w641 w729 w847 w1008 w1060 w1105 w1151 w1194 w1233 w1265 w1298 w1340 w1428 w1549 w1608 w1655 w1717 w1778 w1872 w1954 w2005] -> w207
      tunnel: [w259 w297 w335 w366 w481 w644 w732 w850 w1011 w1052 w1097 w1145 w1189 w1229 w1260 w1297 w1357 w1427 w1548 w1597 w1654 w1716 w1777 w1871 w1953 w1997] -> w68
      tunnel: w206 -> [_ _ _ _ w483 w648 w737 w852 w1015 _ _ _ _ _ _ _ _ w1424 w1545 _ w1653 w1715 w1776 w1843 w1929 _]
      tunnel: "Gate" -> [_ _ _ _ w461 w632 w711 w830 w990 _ _ _ _ _ _ _ _ _ _ _ _ _ _ _ _ _]
      tunnel: "Drain 2" -> [_ _ _ _ w460 w631 w710 w829 w989 _ _ _ _ _ _ _ _ _ _ _ _ _ _ _ _ _]
      tunnel: "Panel Controls" -> [_ _ _ _ _ _ w709 w756 w988 _ _ _ _ _ _ _ _ _ _ _ _ _ _ _ _ _]
      tunnel: w202 -> [w253 w291 w331 w358 w445 w622 w694 w814 w974 w1059 w1104 _ w1187 w1227 w1258 w1296 w1341 w1415 w1536 w1602 w1643 w1705 w1766 w1866 w1948 w2006]
      tunnel: w201 -> [w252 w290 w330 w357 w444 w621 w693 w813 w973 w1058 w1103 w1150 _ w1218 w1264 w1295 w1342 w1416 w1537 w1603 w1644 w1706 w1767 w1867 w1949 w2007]
      tunnel: w200 -> [w251 w289 w329 w356 w443 w620 w692 w812 w972 w1057 w1102 w1149 w1193 w1232 _ w1294 w1343 w1417 w1538 w1604 w1645 w1707 w1768 w1868 w1950 w2008]
      tunnel: w199 -> [w250 w288 w328 w355 w442 w619 w691 w811 w975 w1056 w1101 w1148 w1192 _ w1263 w1293 w1344 w1418 w1539 w1605 w1646 w1708 w1769 w1869 w1951 w2009]
      tunnel: [w253 w291 w331 w358 w445 w622 w694 w814 w974 w1059 w1104 w1143 w1187 w1227 w1258 w1296 w1341 w1415 w1536 w1602 w1643 w1705 w1766 w1866 w1948 w2006] -> w198
      tunnel: [w252 w290 w330 w357 w444 w621 w693 w813 w973 w1058 w1103 w1150 w1179 w1218 w1264 w1295 w1342 w1416 w1537 w1603 w1644 w1706 w1767 w1867 w1949 w2007] -> w197
      tunnel: [w251 w289 w329 w356 w443 w620 w692 w812 w972 w1057 w1102 w1149 w1193 w1232 w1257 w1294 w1343 w1417 w1538 w1604 w1645 w1707 w1768 w1868 w1950 w2008] -> w196
      tunnel: [w250 w288 w328 w355 w442 w619 w691 w811 w975 w1056 w1101 w1148 w1192 w1219 w1263 w1293 w1344 w1418 w1539 w1605 w1646 w1708 w1769 w1869 w1951 w2009] -> w195
      tunnel: w194 -> [w234 w269 w306 _ w383 w574 w663 w752 w943 w1032 w1080 w1127 w1163 w1202 w1241 w1277 w1307 w1402 w1502 w1581 w1614 w1680 w1742 w1802 w1888 w1966]
      tunnel: w193 -> [_ _ _ _ w436 w616 _ _ _ _ _ _ _ _ _ _ _ _ _ _ _ _ _ _ _ _]
      tunnel: [w249 w284 w321 w370 w398 w593 w681 w768 w961 w1051 w1095 w1142 w1178 w1217 w1256 w1292 w1325 w1392 w1506 w1596 w1632 w1698 w1760 w1820 w1906 w1998] -> w111
      tunnel: w192 -> [w249 w284 w321 w370 w433 w593 w681 w803 w961 w1051 w1095 w1142 w1178 w1217 w1256 w1292 w1325 w1398 w1506 w1596 w1632 w1698 w1760 w1820 w1906 w1998]
      tunnel: w92 -> [_ _ _ _ w432 w590 w679 w802 w958 _ _ _ _ _ _ _ w1323 w1407 w1518 _ w1629 w1695 w1757 w1817 w1902 _]
      tunnel: w190 -> [_ _ _ _ w429 w589 w677 w799 w957 _ _ _ _ _ _ _ w1321 w1405 w1517 _ w1628 w1694 w1756 w1816 w1903 _]
      tunnel: w93 -> [_ _ _ _ w425 _ _ w795 _ _ _ _ _ _ _ _ _ _ _ _ _ _ _ _ _ _]
      tunnel: [w248 w283 w320 w360 w402 w592 w680 w772 w960 w1050 w1094 w1141 w1177 w1216 w1255 w1291 w1324 w1377 w1520 w1595 w1631 w1697 w1759 w1819 w1905 w2004] -> w146
      tunnel: w188 -> [w248 w283 w320 w360 w428 w592 w680 w798 w960 w1050 w1094 w1141 w1177 w1216 w1255 w1291 w1324 w1379 w1520 w1595 w1631 w1697 w1759 w1819 w1905 w2004]
      tunnel: [w247 w282 w319 w369 w397 w588 w676 w767 w956 w1049 w1093 w1140 w1176 w1215 w1254 w1290 w1320 w1391 w1505 w1594 w1627 w1693 w1755 w1815 w1901 w1993] -> w110
      tunnel: w164 -> [w247 w282 w319 w369 w424 w588 w676 w794 w956 w1049 w1093 w1140 w1176 w1215 w1254 w1290 w1320 w1397 w1505 w1594 w1627 w1693 w1755 w1815 w1901 w1993]
      tunnel: [w246 w281 w318 w354 w417 w587 w675 w787 w955 w1048 w1092 w1139 w1175 w1214 w1253 w1289 w1319 w1404 w1516 w1593 w1626 w1692 w1754 w1814 w1900 w1992] -> w141
      tunnel: w151 -> [w246 w281 w318 w354 w417 w587 w675 w787 w955 w1048 w1092 w1139 w1175 w1214 w1253 w1289 w1319 w1404 w1516 w1593 w1626 w1692 w1754 w1814 w1900 w1991]
      tunnel: [w245 w280 w317 w363 w416 w586 w674 w786 w954 w1047 w1091 w1138 w1174 w1213 w1252 w1288 w1318 w1403 w1515 w1592 w1625 w1691 w1753 w1813 w1899 w1977] -> w142
      tunnel: w144 -> [w245 w280 w317 w363 w416 w586 w674 w786 w954 w1047 w1091 w1138 w1174 w1213 w1252 w1288 w1318 w1403 w1515 w1592 w1625 w1691 w1753 w1813 w1899 w1977]
      tunnel: [w243 w278 w315 w375 w391 w583 w672 w761 w952 w1045 w1090 w1137 w1172 w1211 w1250 w1286 w1316 w1385 w1514 w1591 w1624 w1690 w1751 w1812 w1898 w1976] -> w104
      tunnel: w132 -> [w243 w278 w315 w375 w415 w583 w672 w785 w952 w1045 w1090 w1137 w1172 w1211 w1250 w1286 w1316 w1385 w1514 w1591 w1624 w1690 w1751 w1812 w1898 w1976]
      tunnel: [w244 w279 w316 w376 w392 w584 w673 w762 w953 w1046 w1089 w1136 w1173 w1212 w1251 w1287 w1317 w1386 w1513 w1590 w1623 w1689 w1752 w1811 w1897 w1975] -> w105
      tunnel: w131 -> [w244 w279 w316 w376 w414 w584 w673 w784 w953 w1046 w1089 w1136 w1173 w1212 w1251 w1287 w1317 w1386 w1513 w1590 w1623 w1689 w1752 w1811 w1897 w1975]
      tunnel: [w236 w271 w308 w368 w396 w580 w670 w766 w950 w1038 w1087 w1134 w1170 w1209 w1248 w1284 w1309 w1390 w1504 w1589 w1616 w1682 w1744 w1804 w1892 w1968] -> w109
      tunnel: w120 -> [w236 w271 w308 w368 w410 w580 w670 w780 w950 w1038 w1087 w1134 w1170 w1209 w1248 w1284 w1309 w1396 w1504 w1589 w1616 w1682 w1744 w1804 w1892 w1968]
      tunnel: [w235 w270 w307 w367 w395 w581 w671 w765 w951 w1037 w1088 w1135 w1171 w1210 w1249 w1285 w1308 w1389 w1503 w1588 w1615 w1681 w1743 w1803 w1891 w1967] -> w108
      tunnel: w119 -> [w235 w270 w307 w367 w409 w581 w671 w779 w951 w1037 w1088 w1135 w1171 w1210 w1249 w1285 w1308 w1395 w1503 w1588 w1615 w1681 w1743 w1803 w1891 w1967]
      tunnel: [w238 w273 w310 w372 w401 w579 w668 w771 w948 w1043 w1085 w1132 w1168 w1207 w1246 w1282 w1311 w1394 w1508 w1583 w1618 w1684 w1746 w1806 w1890 w1972] -> w102
      tunnel: w118 -> [w238 w273 w310 w372 w408 w579 w668 w778 w948 w1043 w1085 w1132 w1168 w1207 w1246 w1282 w1311 w1400 w1508 w1583 w1618 w1684 w1746 w1806 w1890 w1972]
      tunnel: [w237 w272 w309 w371 w399 w582 w669 w769 w949 w1044 w1086 w1133 w1169 w1208 w1247 w1283 w1310 w1393 w1507 w1582 w1617 w1683 w1745 w1805 w1889 w1971] -> w112
      tunnel: w117 -> [w237 w272 w309 w371 w407 w582 w669 w777 w949 w1044 w1086 w1133 w1169 w1208 w1247 w1283 w1310 w1399 w1507 w1582 w1617 w1683 w1745 w1805 w1889 w1971]
      tunnel: [w240 w275 w312 w374 w390 w578 w666 w760 w946 w1041 w1083 w1130 w1166 w1205 w1244 w1280 w1313 w1384 w1510 w1585 w1620 w1686 w1748 w1808 w1894 w1974] -> w103
      tunnel: w116 -> [w240 w275 w312 w374 w406 w578 w666 w776 w946 w1041 w1083 w1130 w1166 w1205 w1244 w1280 w1313 w1384 w1510 w1585 w1620 w1686 w1748 w1808 w1894 w1974]
      tunnel: [w239 w274 w311 w373 w389 w577 w667 w759 w947 w1042 w1084 w1131 w1167 w1206 w1245 w1281 w1312 w1383 w1509 w1584 w1619 w1685 w1747 w1807 w1893 w1973] -> w101
      tunnel: w115 -> [w239 w274 w311 w373 w405 w577 w667 w775 w947 w1042 w1084 w1131 w1167 w1206 w1245 w1281 w1312 w1383 w1509 w1584 w1619 w1685 w1747 w1807 w1893 w1973]
      tunnel: [w242 w277 w314 w378 w394 w576 w664 w764 w944 w1039 w1081 w1128 w1164 w1203 w1242 w1278 w1315 w1388 w1512 w1587 w1622 w1688 w1750 w1810 w1896 w1970] -> w107
      tunnel: w114 -> [w242 w277 w314 w378 w404 w576 w664 w774 w944 w1039 w1081 w1128 w1164 w1203 w1242 w1278 w1315 w1388 w1512 w1587 w1622 w1688 w1750 w1810 w1896 w1970]
      tunnel: [w241 w276 w313 w377 w393 w575 w665 w763 w945 w1040 w1082 w1129 w1165 w1204 w1243 w1279 w1314 w1387 w1511 w1586 w1621 w1687 w1749 w1809 w1895 w1969] -> w106
      tunnel: w113 -> [w241 w276 w313 w377 w403 w575 w665 w773 w945 w1040 w1082 w1129 w1165 w1204 w1243 w1279 w1314 w1387 w1511 w1586 w1621 w1687 w1749 w1809 w1895 w1969]
      tunnel: [w234 w269 w306 w344 w383 w574 w663 w752 w943 w1032 w1080 w1127 w1163 w1202 w1241 w1277 w1307 w1402 w1502 w1581 w1614 w1680 w1742 w1802 w1888 w1966] -> w94
      tunnel: w92 -> [_ _ _ _ _ _ _ _ _ _ _ _ _ _ _ _ _ w1373 _ _ _ _ _ _ _ _]
      tunnel: [w233 w268 w305 w343 w382 w573 w662 w751 w942 w1031 w1079 w1126 w1162 w1201 w1240 w1276 w1306 w1364 w1501 w1580 w1613 w1679 w1741 w1801 w1887 w1965] -> w64
      tunnel: [w232 w267 w304 w342 w381 w572 w661 w750 w941 w1030 w1078 w1125 w1161 w1200 w1239 w1275 w1305 w1361 w1500 w1579 w1612 w1678 w1740 w1800 w1886 w1964] -> w65
      tunnel: [w231 w266 w303 w341 w380 w571 w660 w749 w940 w1029 w1077 w1124 w1160 w1199 w1238 w1274 w1304 w1362 w1499 w1578 w1611 w1677 w1739 w1799 w1885 w1963] -> w66
      tunnel: [w230 w265 w302 w340 w379 w570 w659 w748 w939 w1028 w1076 w1123 w1159 w1198 w1237 w1273 w1303 w1363 w1498 w1577 w1610 w1676 w1738 w1798 w1884 w1962] -> w67
      tunnel: w91 -> [w233 w268 w305 w343 w382 w573 w662 w751 w942 w1031 w1079 w1126 w1162 w1201 w1240 w1276 w1306 w1368 w1501 w1580 w1613 w1679 w1741 w1801 w1887 w1965]
      tunnel: w90 -> [w232 w267 w304 w342 w381 w572 w661 w750 w941 w1030 w1078 w1125 w1161 w1200 w1239 w1275 w1305 w1367 w1500 w1579 w1612 w1678 w1740 w1800 w1886 w1964]
      tunnel: w89 -> [w231 w266 w303 w341 w380 w571 w660 w749 w940 w1029 w1077 w1124 w1160 w1199 w1238 w1274 w1304 w1366 w1499 w1578 w1611 w1677 w1739 w1799 w1885 w1963]
      tunnel: w88 -> [w230 w265 w302 w340 w379 w570 w659 w748 w939 w1028 w1076 w1123 w1159 w1198 w1237 w1273 w1303 w1365 w1498 w1577 w1610 w1676 w1738 w1798 w1884 w1962]
      frame "wait" {
        n33 = Index Array(array=w264, index=0 ("Index")) -> (element=w262:string)
        n34 = Decimal String To Number(string=w262, default (0L)=u32 0) -> (number=w261:u32)  [unwired: 1 in, 1 out]
        n35 = Wait (ms)(milliseconds to wait=w261) -> ()  [unwired: 1 out]
      }
      frame "wait-min" {
        n36 = Index Array(array=w301, index=0 ("Index")) -> (element=w299:string)
        n37 = Decimal String To Number(string=w299, default (0L)=u32 0) -> (number=w287:u32)  [unwired: 1 in, 1 out]
        n38 = Multiply(x=w287, y=u32 60000) -> (x*y=w286:u32)
        n39 = Wait (ms)(milliseconds to wait=w286) -> ()  [unwired: 1 out]
      }
      frame "standby" {
        n40 = Index Array(array=w337, index=0 ("Index")) -> (element=w327:string)
        n41 = case shown="\"off\", Default" w327 {
          tunnel: [":PAGE:SCON:STAN 0" ":PAGE:SCON:STAN 1"] -> w322
          frame "off", Default {
          }
          frame "on" {
          }
        }
        n42 = VISA Write(VISA resource name=w326, write buffer=w322, error in (no error)=w325) -> (VISA resource name out=w324:refnum<visa-resource-name>, error out=w323:errorcluster)  [unwired: 1 out]
      }
      frame "SMU4" {
        n43 = Delete From Array(array=w353, index=0) -> (deleted portion=w347:string, array with subset deleted=w350:string[])  [unwired: 1 in]
        n44 = Equal?(x=w347, y="ON") -> (x = y?=w345:bool)
        n45 = Delete From Array(array=w350, index=0) -> (deleted portion=w349:string)  [unwired: 1 in, 1 out]
        n46 = Fract/Exp String To Number(string=w349) -> (number=w346:dbl)  [unwired: 3 in, 1 out]
        n47 = Bundle(w345, w346) -> (w344:cluster{bool, dbl})  [unwired: 1 in]
      }
      frame "transfer" {
        n48 = Delete From Array(array=w474, index=0 ("Index")) -> (deleted portion=w472:string, array with subset deleted=w471:string[])  [unwired: 1 in]
        n49 = Bundle By Name(cluster=w436, "Emergency Stop"=w483) -> (w437:T2)
        n50 = Number To Decimal String(number=w432) -> (decimal integer string=w431:string)  [unwired: 1 in]
        n51 = case shown="\"d\", Default" w472 {
          tunnel: [w568 w569] -> w470
          frame "s" {
            w568 = u16 0 items=["Single", "Double"] ("sweep mode")
          }
          frame "d", Default {
            w569 = u16 1 items=["Single", "Double"] ("sweep mode")
          }
        }
        n52 = Fract/Exp String To Number(string=w471) -> (number=w456:dbl[])  [unwired: 3 in, 1 out]
        n53 = Concatenate Strings(w481, "-transfer-" ("Prefix"), w431, w429, ".txt" ("Suffix (transfer)")) -> (w482:string)
        n54 = VISA Write(VISA resource name=w452, write buffer=":PAGE:CHAN:MODE SWE;" ("write buffer (\"\")"), error in (no error)=w451) -> (VISA resource name out=w449:refnum<visa-resource-name>, error out=w450:errorcluster)  [unwired: 1 out]
        n55 = local read "Plot transfer curve extrema vs time"() -> (w384:bool)
        n56 = String To Path(string=w482) -> (path=w480:path)
        n57 = Index Array(array=w456, index #1=0 ("Index")) -> (element #1=w469:dbl, element #2=w468:dbl, element #3=w467:dbl)  [unwired: 2 in]
        n58 = Delete From Array(array=w456, length=3 ("Length"), index=0 ("Index")) -> (array with subset deleted=w454:dbl[])  [unwired: 1 out]
        n59 = case shown="True" w384 {
          tunnel: w428 -> [w485 w488]
          tunnel: w425 -> [_ w487]
          tunnel: [w485 w486] -> w402
          frame False {
          }
          frame True {
            n60 = Build Array (concatenate)(w488, w487) -> (w486:i32[])
          }
        }
        n61 = Bundle By Name(cluster=w461, "Gate Start"=w469, "Gate Stop"=w468, "Gate Step (linear only)"=w467, "Gate Compliance"=w478, "Range mode"=w445, "Range"=w444) -> (w446:T6)
        n62 = Index Array(array=w454, index #1=0 ("Index")) -> (element #1=w464:dbl, element #2=w463:dbl, element #3=w462:dbl)  [unwired: 2 in]
        n63 = call <vilib>:"compatOverwrite.vi"("overwrite (F)"=TRUE) -> ("overwrite?"=w435:T8)
        n64 = Bundle By Name(cluster=w460, "Drain Start"=w464, "Drain Stop"=w463, "Drain Step"=w462, "Drain Compliance"=w479, "Range mode"=w443, "Range"=w442) -> (w447:T7)
        n65 = call "4155C Transfer.vi"("VISA resource name in"=w449, "Gate"=w446, "Drain"=w447, "Timings"=w477, "error in (no error)"=w450, "SMU4"=w383, "sweep mode"=w470, "Panel Controls"=w437) -> ("VG"=w434:dbl[], "Outparams"=w441:T9, "VISA Resource Name out"=w476:refnum<visa-resource-name>, "IS"=w412:dbl[], "ID"=w413:dbl[], "IG"=w411:dbl[], "error out"=w426:errorcluster, "SMU4"=w438:dbl[])  [unwired: 12 in]
        n66 = Unbundle By Name(w441) -> ("V2 Step"=w440:dbl, "V2 Start"=w439:dbl, "Number of points"=w400:i32)
        n67 = call "4155C Split array.vi"("Number of VAR2 steps"=w400, "Y2 data in"=w413, "X data in"=w434, "Y1 data in"=w412, "Y3 data in"=w411, "error in (no error)"=w426) -> ("Array of clusters"=w427:cluster{"Y data in":dbl[], "X data in":dbl[]}[], "error out"=w388:errorcluster)  [unwired: 1 in]
        n68 = case shown="True" "Plot transfer curve extrema vs time" {
          tunnel: w433 -> [w491 w567]
          tunnel: w424 -> [w492 w562]
          tunnel: w415 -> [w498 w558]
          tunnel: w414 -> [w499 w557]
          tunnel: w413 -> [_ w554]
          tunnel: w412 -> [_ w552]
          tunnel: w411 -> [_ w551]
          tunnel: w410 -> [w493 w547]
          tunnel: w409 -> [w495 w546]
          tunnel: w408 -> [w489 w543]
          tunnel: w407 -> [w490 w542]
          tunnel: w406 -> [w497 w539]
          tunnel: w405 -> [w496 w538]
          tunnel: w404 -> [w501 w535]
          tunnel: w403 -> [w500 w534]
          tunnel: w402 -> [_ w527]
          tunnel: [w489 w522] -> w401
          tunnel: w400 -> [_ w521]
          tunnel: [w490 w520] -> w399
          tunnel: [w491 w519] -> w398
          tunnel: [w492 w518] -> w397
          tunnel: [w493 w517] -> w396
          tunnel: [w495 w516] -> w395
          tunnel: [w501 w515] -> w394
          tunnel: [w500 w514] -> w393
          tunnel: [w499 w513] -> w392
          tunnel: [w498 w512] -> w391
          tunnel: [w497 w511] -> w390
          tunnel: [w496 w510] -> w389
          tunnel: w388 -> [w494 w509]
          tunnel: [w494 w505] -> w387
          frame False {
          }
          frame True {
            # "Adjusts graph colors."
            # "Adjusts graph colors."
            # "Ion will be the middle element of the array. The calculation of the index is done only once, since Is, Id, and Ig have the same dimensions."
            # "abs(Ig)"
            # "abs(Is)"
            # "Y1: Is\nY2: Id\nY3: Ig"
            # "abs(Id)"
            # "Adjusts graph colors."
            # "Adjusts graph colors."
            # "Adjusts graph colors."
            n69 = Absolute Value(x=w552) -> (abs(x)=w537:dbl[])
            n70 = Absolute Value(x=w554) -> (abs(x)=w553:dbl[])
            n71 = Absolute Value(x=w551) -> (abs(x)=w540:dbl[])
            n72 = Array Size(array=w553) -> (size(s)=w561:i32)
            n73 = Divide(x=w561, y=2) -> (x/y=w504:dbl)
            n74 = Subtract(x=w504, y=1) -> (x-y=w503:dbl)
            n75 = Array Max & Min(array=w537) -> (max value=w544:dbl, min value=w545:dbl)  [unwired: 2 out]
            n76 = Array Max & Min(array=w553) -> (max value=w566:dbl, min value=w550:dbl)  [unwired: 2 out]
            n77 = Array Max & Min(array=w540) -> (max value=w549:dbl, min value=w548:dbl)  [unwired: 2 out]
            n78 = Index Array(array=w537, index=w503) -> (element=w528:dbl)
            n79 = Index Array(array=w537, index=0) -> (element=w529:dbl)
            n80 = Index Array(array=w553, index=w503) -> (element=w530:dbl)
            n81 = Index Array(array=w553, index=0) -> (element=w531:dbl)
            n82 = Index Array(array=w540, index=w503) -> (element=w533:dbl)
            n83 = Index Array(array=w540, index=0) -> (element=w532:dbl)
            n84 = local write "Ig max"(w549) -> ()
            n85 = local write "Ig min"(w548) -> ()
            n86 = local write "Is max"(w544) -> ()
            n87 = local write "Is min"(w545) -> ()
            n88 = local write "Id max"(w566) -> ()
            n89 = local write "Id min"(w550) -> ()
            n90 = Build Array (concatenate)(w543, w544) -> (w522:dbl[])
            n91 = Build Array (concatenate)(w542, w545) -> (w520:dbl[])
            n92 = local write "Is off"(w529) -> ()
            n93 = local write "Is on"(w528) -> ()
            n94 = Build Array (concatenate)(w567, w566) -> (w519:dbl[])
            n95 = Build Array (concatenate)(w562, w550) -> (w518:dbl[])
            n96 = Build Array (concatenate)(w547, w549) -> (w517:dbl[])
            n97 = Build Array (concatenate)(w546, w548) -> (w516:dbl[])
            n98 = Build Array (concatenate)(w535, w528) -> (w515:dbl[])
            n99 = Build Array (concatenate)(w534, w529) -> (w514:dbl[])
            n100 = Build Array (concatenate)(w557, w530) -> (w513:dbl[])
            n101 = Build Array (concatenate)(w558, w531) -> (w512:dbl[])
            n102 = Build Array (concatenate)(w539, w533) -> (w511:dbl[])
            n103 = Build Array (concatenate)(w538, w532) -> (w510:dbl[])
            n104 = local write "Ig off"(w532) -> ()
            n105 = local write "Ig on"(w533) -> ()
            n106 = local write "Id off"(w531) -> ()
            n107 = local write "Id on"(w530) -> ()
            n108 = control-ref of="Imax vs time"() -> (w556:refnum<vi>)
            n109 = control-ref of="Imin vs time"() -> (w555:refnum<vi>)
            n110 = control-ref of="Ion vs time"() -> (w524:refnum<vi>)
            n111 = control-ref of="Ioff vs time"() -> (w523:refnum<vi>)
            n112 = control-ref of="I vs Vg"() -> (w565:refnum<vi>)
            n113 = call "4155C Split array.vi"("Number of VAR2 steps"=w521, "Y2 data in"=w513, "X data in"=w527, "Y1 data in"=w515, "Y3 data in"=w511, "error in (no error)"=w509) -> ("Array of clusters"=w525:cluster{"Y data in":dbl[], "X data in":dbl[]}[], "error out"=w508:errorcluster)  [unwired: 1 in]
            n114 = call "4155C Split array.vi"("Number of VAR2 steps"=w521, "Y2 data in"=w512, "X data in"=w527, "Y1 data in"=w514, "Y3 data in"=w510, "error in (no error)"=w508) -> ("Array of clusters"=w526:cluster{"Y data in":dbl[], "X data in":dbl[]}[], "error out"=w507:errorcluster)  [unwired: 1 in]
            n115 = call "4155C Split array.vi"("Number of VAR2 steps"=w521, "Y2 data in"=w519, "X data in"=w527, "Y1 data in"=w522, "Y3 data in"=w517, "error in (no error)"=w507) -> ("Array of clusters"=w564:cluster{"Y data in":dbl[], "X data in":dbl[]}[], "error out"=w506:errorcluster)  [unwired: 1 in]
            n116 = call "4155C Split array.vi"("Number of VAR2 steps"=w521, "Y2 data in"=w518, "X data in"=w527, "Y1 data in"=w520, "Y3 data in"=w516, "error in (no error)"=w506) -> ("Array of clusters"=w563:cluster{"Y data in":dbl[], "X data in":dbl[]}[], "error out"=w505:errorcluster)  [unwired: 1 in]
            n117 = call "4155C Config Chart Colours.vi"("Numeric"=w521, "XY Graph 2"=w556) -> ()  [unwired: 6 in]
            n118 = call "4155C Config Chart Colours.vi"("Numeric"=w521, "XY Graph 2"=w555) -> ()  [unwired: 6 in]
            n119 = call "4155C Config Chart Colours.vi"("Numeric"=w521, "XY Graph 2"=w524) -> ()  [unwired: 6 in]
            n120 = call "4155C Config Chart Colours.vi"("Numeric"=w521, "XY Graph 2"=w523) -> ()  [unwired: 6 in]
            n121 = call "4155C Config Chart Colours.vi"("Numeric"=w521, "XY Graph 2"=w565) -> ()  [unwired: 6 in]
            n122 = local write "Imax vs time"(w564) -> ()
            n123 = local write "Imin vs time"(w563) -> ()
            n124 = local write "Ion vs time"(w525) -> ()
            n125 = local write "Ioff vs time"(w526) -> ()
          }
        }
        n126 = local write "I vs Vg"(w427) -> ()
        n127 = Open/Create/Replace File(file path (use dialog)=w480, error in=w387, operation (0:open)=w435) -> (refnum out=w422:refnum<file>, error out=w420:errorcluster)  [unwired: 3 in, 1 out]
        n128 = call "4155C Make Big 2d array.vi"("1D Var1"=w434, "1d IS"=w412, "1d ID"=w413, "1d IG"=w411, "1d SMU4"=w438, "SMU4"=w383, "VAR2 START"=w439, "Number of VAR2 steps"=w400, "VAR2 STEP"=w440, "VAR1 Name"="Vg", "Decimal places in header"=i8 1, "VAR2 Name"="Vd") -> ("Header array"=w423:string[], "Data array"=w421:dbl[][])  [unwired: 14 in]
        n129 = call "4155C Write array to file.vi"("Byte Stream File Refnum"=w422, "Header"=w423, "Data Array"=w421, "error in (no error)"=w420) -> ("dup refnum"=w419:refnum<file>, "error out"=w418:errorcluster)  [unwired: 1 in]
        n130 = Close File(refnum=w419, error in=w418) -> (error out=w475:errorcluster)  [unwired: 1 out]
      }
      frame "pulsedstressV" {
        w599 = 0
        n131 = Number To Decimal String(number=w590) -> (decimal integer string=w645:string)  [unwired: 1 in]
        n132 = Delete From Array(array=w585, index=0 ("Index")) -> (deleted portion=w636:string, array with subset deleted=w635:string[])  [unwired: 1 in]
        n133 = Bundle By Name(cluster=w616, "Emergency Stop"=w648) -> (w617:T2)
        n134 = VISA Write(VISA resource name=w629, write buffer=":PAGE:CHAN:MODE SWE;" ("write buffer (\"\")"), error in (no error)=w628) -> (VISA resource name out=w626:refnum<visa-resource-name>, error out=w627:errorcluster)  [unwired: 1 out]
        n135 = Concatenate Strings(w644, "-pulsedstressV-" ("Substring"), w645, w589, ".txt" ("Substring")) -> (w647:string)
        n136 = case shown="\"d\", Default" w636 {
          tunnel: [w657 w658] -> w634
          frame "s" {
            w657 = u16 0 items=["Single", "Double"] ("sweep mode")
          }
          frame "d", Default {
            w658 = u16 1 items=["Single", "Double"] ("sweep mode")
          }
        }
        n137 = Fract/Exp String To Number(string=w635) -> (number=w630:dbl[])  [unwired: 3 in, 1 out]
        n138 = String To Path(string=w647) -> (path=w643:path)
        n139 = Index Array(array=w630, index #1=0 ("Index")) -> (element #1=w608:dbl, element #2=w607:dbl, element #3=w604:dbl, element #4=w603:dbl, element #5=w602:dbl, element #6=w606:dbl)  [unwired: 5 in]
        n140 = Bundle By Name(cluster=w605, "Pulse period"=w603, "Base voltage"=w604, "Pulse width"=w602) -> (w601:T4)
        n141 = Unbundle By Name(w601) -> ("Pulse period"=w609:dbl)
        n142 = Bundle By Name(cluster=w632, "Gate Start"=w607, "Gate Stop"=w608, "Gate Step (linear only)"=0, "Gate Compliance"=w641, "Range mode"=w622, "Range"=w621) -> (w623:T6)
        n143 = call <vilib>:"compatOverwrite.vi"("overwrite (F)"=TRUE) -> ("overwrite?"=w594:T8)
        n144 = Bundle By Name(cluster=w631, "Drain Start"=w606, "Drain Stop"=w599, "Drain Step"=w599, "Drain Compliance"=w642, "Range mode"=w620, "Range"=w619) -> (w624:T7)
        n145 = call "4155C PulsedStressV.vi"("VISA resource name in"=w626, "sweep mode"=w634, "Panel Controls"=w617, "Gate"=w623, "Drain"=w624, "Timings"=w601, "error in (no error)"=w627, "SMU4"=w574) -> ("VISA Resource Name out"=w639:refnum<visa-resource-name>, "ID"=w597:dbl[], "IG"=w595:dbl[], "Outparams"=w618:T9, "error out"=w640:errorcluster)  [unwired: 3 in]
        n146 = Unbundle By Name(w618) -> ("Number of points"=w596:i32)  [unwired: 2 out]
        n147 = for {
          N: w596 -> [_]
          tunnel: [w654] -> w598 mode=indexing
          tunnel: w609 -> [w656]
          i -> [w655]
          n148 = Multiply(x=w656, y=w655) -> (x*y=w654:dbl)
        }
        n149 = Insert Into Array(array=dbl[][] [] ("Input Array"), new element=w598) -> (w610:dbl[][])  [unwired: 2 in]
        n150 = Insert Into Array(array=w610, new element=w597) -> (w615:dbl[][])  [unwired: 2 in]
        n151 = Insert Into Array(array=w615, new element=w595) -> (w614:dbl[][])  [unwired: 2 in]
        n152 = Transpose 2D Array(2D array=w614) -> (transposed array=w613:dbl[][])
        n153 = Open/Create/Replace File(file path (use dialog)=w643, error in=w640, operation (0:open)=w594) -> (refnum out=w651:refnum<file>, error out=w652:errorcluster)  [unwired: 3 in, 1 out]
        n154 = call "4155C Write array to file.vi"("Byte Stream File Refnum"=w651, "Header"=string[] ["Time /s", "Id /A", "Ig /A"], "Data Array"=w613, "error in (no error)"=w652) -> ("dup refnum"=w649:refnum<file>, "error out"=w650:errorcluster)  [unwired: 1 in]
        n155 = Close File(refnum=w649, error in=w650) -> (error out=w638:errorcluster)  [unwired: 1 out]
      }
      frame "transfer-fpp" {
        n156 = Number To Decimal String(number=w679) -> (decimal integer string=w733:string)  [unwired: 1 in]
        n157 = Bundle By Name(cluster=w709, "Emergency Stop"=w737) -> (w745:T1)
        n158 = Delete From Array(array=w724, index=0 ("Index")) -> (deleted portion=w722:string, array with subset deleted=w721:string[])  [unwired: 1 in]
        n159 = Concatenate Strings(w732, "-transferfpp-" ("Substring"), w733, w677, ".txt" ("Substring")) -> (w735:string)
        n160 = VISA Write(VISA resource name=w701, write buffer=":PAGE:CHAN:MODE SWE;" ("write buffer (\"\")"), error in (no error)=w700) -> (VISA resource name out=w698:refnum<visa-resource-name>, error out=w699:errorcluster)  [unwired: 1 out]
        n161 = case shown="\"d\", Default" w722 {
          tunnel: [w746 w747] -> w720
          frame "s" {
            w746 = u16 0 items=["Single", "Double"] ("sweep mode")
          }
          frame "d", Default {
            w747 = u16 1 items=["Single", "Double"] ("sweep mode")
          }
        }
        n162 = Fract/Exp String To Number(string=w721) -> (number=w705:dbl[])  [unwired: 3 in, 1 out]
        n163 = String To Path(string=w735) -> (path=w731:path)
        n164 = Index Array(array=w705, index #1=0 ("Index")) -> (element #1=w719:dbl, element #2=w718:dbl, element #3=w717:dbl)  [unwired: 2 in]
        n165 = Delete From Array(array=w705, length=3 ("Length"), index=0 ("Index")) -> (array with subset deleted=w703:dbl[])  [unwired: 1 out]
        n166 = Bundle By Name(cluster=w711, "Gate Start"=w719, "Gate Stop"=w718, "Gate Step (linear only)"=w717, "Gate Compliance"=w729, "Range mode"=w694, "Range"=w693) -> (w695:T6)
        n167 = Index Array(array=w703, index #1=0 ("Index")) -> (element #1=w714:dbl, element #2=w713:dbl, element #3=w712:dbl)  [unwired: 2 in]
        n168 = call <vilib>:"compatOverwrite.vi"("overwrite (F)"=TRUE) -> ("overwrite?"=w682:T8)
        n169 = Bundle By Name(cluster=w710, "Drain Start"=w714, "Drain Stop"=w713, "Drain Step"=w712, "Drain Compliance"=w730, "Range mode"=w692, "Range"=w691) -> (w696:T7)
        n170 = call "4155C Transfer-FPP.vi"("VISA resource name in"=w698, "Gate"=w695, "Drain"=w696, "Timings"=w728, "error in (no error)"=w699, "sweep mode"=w720, "Panel Controls"=w745) -> ("VG"=w736:dbl[], "Outparams"=w690:T9, "VISA Resource Name out"=w726:refnum<visa-resource-name>, "Vprobe2"=w686:dbl[], "ID"=w685:dbl[], "IG"=w684:dbl[], "Vprobe1"=w683:dbl[], "error out"=w727:errorcluster)  [unwired: 13 in]
        n171 = Unbundle By Name(w690) -> ("V2 Step"=w689:dbl, "V2 Start"=w688:dbl, "Number of points"=w687:i32)
        n172 = Open/Create/Replace File(file path (use dialog)=w731, error in=w727, operation (0:open)=w682) -> (refnum out=w742:refnum<file>, error out=w743:errorcluster)  [unwired: 3 in, 1 out]
        n173 = call "4155C Make Big 2d array FPP.vi"("1D Var1"=w736, "1d ID"=w685, "1d Vp2"=w686, "1d IG"=w684, "1d Vp1"=w683, "VAR2 START"=w688, "Number of VAR2 steps"=w687, "VAR2 STEP"=w689, "VAR1 Name"="Vg", "Decimal places in header"=i8 1, "VAR2 Name"="Vd") -> ("Header array"=w738:string[], "Data array"=w739:dbl[][])  [unwired: 15 in]
        n174 = call "4155C Write array to file.vi"("Byte Stream File Refnum"=w742, "Header"=w738, "Data Array"=w739, "error in (no error)"=w743) -> ("dup refnum"=w740:refnum<file>, "error out"=w741:errorcluster)  [unwired: 1 in]
        n175 = Close File(refnum=w740, error in=w741) -> (error out=w725:errorcluster)  [unwired: 1 out]
      }
      frame "output" {
        n176 = Delete From Array(array=w843, index=0 ("Index")) -> (deleted portion=w841:string, array with subset deleted=w840:string[])  [unwired: 1 in]
        n177 = Bundle By Name(cluster=w756, "Emergency Stop"=w852) -> (w806:T1)
        n178 = Number To Decimal String(number=w802) -> (decimal integer string=w801:string)  [unwired: 1 in]
        n179 = case shown="\"d\", Default" w841 {
          tunnel: [w937 w938] -> w839
          frame "s" {
            w937 = u16 0 items=["Single", "Double"] ("sweep mode")
          }
          frame "d", Default {
            w938 = u16 1 items=["Single", "Double"] ("sweep mode")
          }
        }
        n180 = Fract/Exp String To Number(string=w840) -> (number=w825:dbl[])  [unwired: 3 in, 1 out]
        n181 = Concatenate Strings(w850, "-output-" ("Substring"), w801, w799, ".txt" ("Suffix (transfer)")) -> (w851:string)
        n182 = VISA Write(VISA resource name=w821, write buffer=":PAGE:CHAN:MODE SWE;" ("write buffer (\"\")"), error in (no error)=w820) -> (VISA resource name out=w818:refnum<visa-resource-name>, error out=w819:errorcluster)  [unwired: 1 out]
        n183 = String To Path(string=w851) -> (path=w849:path)
        n184 = local read "Plot output curve extrema vs time"() -> (w753:bool)
        n185 = Index Array(array=w825, index #1=0 ("Index")) -> (element #1=w838:dbl, element #2=w837:dbl, element #3=w836:dbl)  [unwired: 2 in]
        n186 = Delete From Array(array=w825, length=3 ("Length"), index=0 ("Index")) -> (array with subset deleted=w823:dbl[])  [unwired: 1 out]
        n187 = case shown="True" w753 {
          tunnel: w798 -> [w854 w857]
          tunnel: w795 -> [_ w856]
          tunnel: [w854 w855] -> w772
          frame False {
          }
          frame True {
            n188 = Build Array (concatenate)(w857, w856) -> (w855:i32[])
          }
        }
        n189 = Bundle By Name(cluster=w830, "Gate Start"=w838, "Gate Stop"=w837, "Gate Step (linear only)"=w836, "Gate Compliance"=w847, "Range mode"=w814, "Range"=w813) -> (w815:T6)
        n190 = Index Array(array=w823, index #1=0 ("Index")) -> (element #1=w833:dbl, element #2=w832:dbl, element #3=w831:dbl)  [unwired: 2 in]
        n191 = call <vilib>:"compatOverwrite.vi"("overwrite (F)"=TRUE) -> ("overwrite?"=w805:T8)
        n192 = Bundle By Name(cluster=w829, "Drain Start"=w833, "Drain Stop"=w832, "Drain Step"=w831, "Drain Compliance"=w848, "Range mode"=w812, "Range"=w811) -> (w816:T7)
        n193 = call "4155C Output.vi"("VISA resource name in"=w818, "Gate"=w815, "Drain"=w816, "Timings"=w846, "error in (no error)"=w819, "SMU4"=w752, "sweep mode"=w839, "Panel controls"=w806) -> ("VD"=w804:dbl[], "Outparams"=w810:T9, "VISA Resource Name out"=w845:refnum<visa-resource-name>, "IS"=w782:dbl[], "ID"=w783:dbl[], "IG"=w781:dbl[], "error out"=w796:errorcluster, "SMU4"=w807:dbl[])  [unwired: 12 in]
        n194 = Unbundle By Name(w810) -> ("V2 Step"=w809:dbl, "V2 Start"=w808:dbl, "Number of points"=w770:i32)
        n195 = call "4155C Split array.vi"("Number of VAR2 steps"=w770, "Y2 data in"=w783, "X data in"=w804, "Y1 data in"=w782, "Y3 data in"=w781, "error in (no error)"=w796) -> ("Array of clusters"=w797:cluster{"Y data in":dbl[], "X data in":dbl[]}[], "error out"=w758:errorcluster)  [unwired: 1 in]
        n196 = case shown="True" "Plot output curve extrema vs time" {
          tunnel: w803 -> [w866 w936]
          tunnel: w794 -> [w867 w931]
          tunnel: w785 -> [w861 w927]
          tunnel: w784 -> [w860 w926]
          tunnel: w783 -> [_ w923]
          tunnel: w782 -> [_ w921]
          tunnel: w781 -> [_ w920]
          tunnel: w780 -> [w868 w916]
          tunnel: w779 -> [w869 w915]
          tunnel: w778 -> [w864 w912]
          tunnel: w777 -> [w865 w911]
          tunnel: w776 -> [w862 w908]
          tunnel: w775 -> [w863 w907]
          tunnel: w774 -> [w858 w904]
          tunnel: w773 -> [w859 w903]
          tunnel: w772 -> [_ w896]
          tunnel: [w864 w891] -> w771
          tunnel: w770 -> [_ w890]
          tunnel: [w865 w889] -> w769
          tunnel: [w866 w888] -> w768
          tunnel: [w867 w887] -> w767
          tunnel: [w868 w886] -> w766
          tunnel: [w869 w885] -> w765
          tunnel: [w858 w884] -> w764
          tunnel: [w859 w883] -> w763
          tunnel: [w860 w882] -> w762
          tunnel: [w861 w881] -> w761
          tunnel: [w862 w880] -> w760
          tunnel: [w863 w879] -> w759
          tunnel: w758 -> [w870 w878]
          tunnel: [w870 w874] -> w757
          frame False {
          }
          frame True {
            # "Adjusts graph colors."
            # "Adjusts graph colors."
            # "Ion will be the middle element of the array. The calculation of the index is done only once, since Is, Id, and Ig have the same dimensions."
            # "abs(Ig)"
            # "abs(Is)"
            # "Y1: Is\nY2: Id\nY3: Ig"
            # "abs(Id)"
            # "Adjusts graph colors."
            # "Adjusts graph colors."
            # "Adjusts graph colors."
            n197 = Absolute Value(x=w921) -> (abs(x)=w906:dbl[])
            n198 = Absolute Value(x=w923) -> (abs(x)=w922:dbl[])
            n199 = Absolute Value(x=w920) -> (abs(x)=w909:dbl[])
            n200 = Array Size(array=w922) -> (size(s)=w930:i32)
            n201 = Divide(x=w930, y=2) -> (x/y=w873:dbl)
            n202 = Subtract(x=w873, y=1) -> (x-y=w872:dbl)
            n203 = Array Max & Min(array=w906) -> (max value=w913:dbl, min value=w914:dbl)  [unwired: 2 out]
            n204 = Array Max & Min(array=w922) -> (max value=w935:dbl, min value=w919:dbl)  [unwired: 2 out]
            n205 = Array Max & Min(array=w909) -> (max value=w918:dbl, min value=w917:dbl)  [unwired: 2 out]
            n206 = Index Array(array=w906, index=w872) -> (element=w897:dbl)
            n207 = Index Array(array=w906, index=0) -> (element=w898:dbl)
            n208 = Index Array(array=w922, index=w872) -> (element=w899:dbl)
            n209 = Index Array(array=w922, index=0) -> (element=w900:dbl)
            n210 = Index Array(array=w909, index=w872) -> (element=w902:dbl)
            n211 = Index Array(array=w909, index=0) -> (element=w901:dbl)
            n212 = local write "Ig max"(w918) -> ()
            n213 = local write "Ig min"(w917) -> ()
            n214 = local write "Is max"(w913) -> ()
            n215 = local write "Is min"(w914) -> ()
            n216 = local write "Id max"(w935) -> ()
            n217 = local write "Id min"(w919) -> ()
            n218 = Build Array (concatenate)(w912, w913) -> (w891:dbl[])
            n219 = Build Array (concatenate)(w911, w914) -> (w889:dbl[])
            n220 = local write "Is off"(w898) -> ()
            n221 = local write "Is on"(w897) -> ()
            n222 = Build Array (concatenate)(w936, w935) -> (w888:dbl[])
            n223 = Build Array (concatenate)(w931, w919) -> (w887:dbl[])
            n224 = Build Array (concatenate)(w916, w918) -> (w886:dbl[])
            n225 = Build Array (concatenate)(w915, w917) -> (w885:dbl[])
            n226 = Build Array (concatenate)(w904, w897) -> (w884:dbl[])
            n227 = Build Array (concatenate)(w903, w898) -> (w883:dbl[])
            n228 = Build Array (concatenate)(w926, w899) -> (w882:dbl[])
            n229 = Build Array (concatenate)(w927, w900) -> (w881:dbl[])
            n230 = Build Array (concatenate)(w908, w902) -> (w880:dbl[])
            n231 = Build Array (concatenate)(w907, w901) -> (w879:dbl[])
            n232 = local write "Ig off"(w901) -> ()
            n233 = local write "Ig on"(w902) -> ()
            n234 = local write "Id off"(w900) -> ()
            n235 = local write "Id on"(w899) -> ()
            n236 = control-ref of="Imax vs time"() -> (w925:refnum<vi>)
            n237 = control-ref of="Imin vs time"() -> (w924:refnum<vi>)
            n238 = control-ref of="Ion vs time"() -> (w893:refnum<vi>)
            n239 = control-ref of="Ioff vs time"() -> (w892:refnum<vi>)
            n240 = control-ref of="I vs Vg"() -> (w934:refnum<vi>)
            n241 = call "4155C Split array.vi"("Number of VAR2 steps"=w890, "Y2 data in"=w882, "X data in"=w896, "Y1 data in"=w884, "Y3 data in"=w880, "error in (no error)"=w878) -> ("Array of clusters"=w894:cluster{"Y data in":dbl[], "X data in":dbl[]}[], "error out"=w877:errorcluster)  [unwired: 1 in]
            n242 = call "4155C Split array.vi"("Number of VAR2 steps"=w890, "Y2 data in"=w881, "X data in"=w896, "Y1 data in"=w883, "Y3 data in"=w879, "error in (no error)"=w877) -> ("Array of clusters"=w895:cluster{"Y data in":dbl[], "X data in":dbl[]}[], "error out"=w876:errorcluster)  [unwired: 1 in]
            n243 = call "4155C Split array.vi"("Number of VAR2 steps"=w890, "Y2 data in"=w888, "X data in"=w896, "Y1 data in"=w891, "Y3 data in"=w886, "error in (no error)"=w876) -> ("Array of clusters"=w933:cluster{"Y data in":dbl[], "X data in":dbl[]}[], "error out"=w875:errorcluster)  [unwired: 1 in]
            n244 = call "4155C Split array.vi"("Number of VAR2 steps"=w890, "Y2 data in"=w887, "X data in"=w896, "Y1 data in"=w889, "Y3 data in"=w885, "error in (no error)"=w875) -> ("Array of clusters"=w932:cluster{"Y data in":dbl[], "X data in":dbl[]}[], "error out"=w874:errorcluster)  [unwired: 1 in]
            n245 = call "4155C Config Chart Colours.vi"("Numeric"=w890, "XY Graph 2"=w925) -> ()  [unwired: 6 in]
            n246 = call "4155C Config Chart Colours.vi"("Numeric"=w890, "XY Graph 2"=w924) -> ()  [unwired: 6 in]
            n247 = call "4155C Config Chart Colours.vi"("Numeric"=w890, "XY Graph 2"=w893) -> ()  [unwired: 6 in]
            n248 = call "4155C Config Chart Colours.vi"("Numeric"=w890, "XY Graph 2"=w892) -> ()  [unwired: 6 in]
            n249 = call "4155C Config Chart Colours.vi"("Numeric"=w890, "XY Graph 2"=w934) -> ()  [unwired: 6 in]
            n250 = local write "Imax vs time"(w933) -> ()
            n251 = local write "Imin vs time"(w932) -> ()
            n252 = local write "Ion vs time"(w894) -> ()
            n253 = local write "Ioff vs time"(w895) -> ()
          }
        }
        n254 = local write "I vs Vd"(w797) -> ()
        n255 = Open/Create/Replace File(file path (use dialog)=w849, error in=w757, operation (0:open)=w805) -> (refnum out=w792:refnum<file>, error out=w790:errorcluster)  [unwired: 3 in, 1 out]
        n256 = call "4155C Make Big 2d array.vi"("1D Var1"=w804, "1d IS"=w782, "1d ID"=w783, "1d IG"=w781, "1d SMU4"=w807, "SMU4"=w752, "VAR2 START"=w808, "Number of VAR2 steps"=w770, "VAR2 STEP"=w809, "VAR1 Name"="Vd", "Decimal places in header"=i8 1, "VAR2 Name"="Vg") -> ("Header array"=w793:string[], "Data array"=w791:dbl[][])  [unwired: 14 in]
        n257 = call "4155C Write array to file.vi"("Byte Stream File Refnum"=w792, "Header"=w793, "Data Array"=w791, "error in (no error)"=w790) -> ("dup refnum"=w789:refnum<file>, "error out"=w788:errorcluster)  [unwired: 1 in]
        n258 = Close File(refnum=w789, error in=w788) -> (error out=w844:errorcluster)  [unwired: 1 out]
      }
      frame "output-fpp" {
        n259 = Number To Decimal String(number=w958) -> (decimal integer string=w1012:string)  [unwired: 1 in]
        n260 = Bundle By Name(cluster=w988, "Emergency Stop"=w1015) -> (w1025:T1)
        n261 = Delete From Array(array=w1003, index=0 ("Index")) -> (deleted portion=w1001:string, array with subset deleted=w1000:string[])  [unwired: 1 in]
        n262 = VISA Write(VISA resource name=w979, write buffer=":PAGE:CHAN:MODE SWE;" ("write buffer (\"\")"), error in (no error)=w976) -> (VISA resource name out=w978:refnum<visa-resource-name>, error out=w977:errorcluster)  [unwired: 1 out]
        n263 = Concatenate Strings(w1011, "-outputfpp-" ("Substring"), w1012, w957, ".txt" ("Substring")) -> (w1014:string)
        n264 = case shown="\"d\", Default" w1001 {
          tunnel: [w1026 w1027] -> w999
          frame "s" {
            w1026 = u16 0 items=["Single", "Double"] ("sweep mode")
          }
          frame "d", Default {
            w1027 = u16 1 items=["Single", "Double"] ("sweep mode")
          }
        }
        n265 = Fract/Exp String To Number(string=w1000) -> (number=w982:dbl[])  [unwired: 3 in, 1 out]
        n266 = String To Path(string=w1014) -> (path=w1010:path)
        n267 = Index Array(array=w982, index #1=0 ("Index")) -> (element #1=w998:dbl, element #2=w997:dbl, element #3=w996:dbl)  [unwired: 2 in]
        n268 = Delete From Array(array=w982, length=3 ("Length"), index=0 ("Index")) -> (array with subset deleted=w981:dbl[])  [unwired: 1 out]
        n269 = Bundle By Name(cluster=w990, "Gate Start"=w998, "Gate Stop"=w997, "Gate Step (linear only)"=w996, "Gate Compliance"=w1008, "Range mode"=w974, "Range"=w973) -> (w1024:T6)
        n270 = Index Array(array=w981, index #1=0 ("Index")) -> (element #1=w993:dbl, element #2=w992:dbl, element #3=w991:dbl)  [unwired: 2 in]
        n271 = call <vilib>:"compatOverwrite.vi"("overwrite (F)"=TRUE) -> ("overwrite?"=w962:T8)
        n272 = Bundle By Name(cluster=w989, "Drain Start"=w993, "Drain Stop"=w992, "Drain Step"=w991, "Drain Compliance"=w1009, "Range mode"=w972, "Range"=w975) -> (w1023:T7)
        n273 = call "4155C Output-FPP.vi"("VISA resource name in"=w978, "Gate"=w1024, "Drain"=w1023, "Timings"=w1007, "error in (no error)"=w977, "sweep mode"=w999, "Panel controls"=w1025) -> ("VD"=w967:dbl[], "Outparams"=w970:T9, "VISA Resource Name out"=w1005:refnum<visa-resource-name>, "Vprobe2"=w966:dbl[], "ID"=w965:dbl[], "IG"=w964:dbl[], "Vprobe1"=w963:dbl[], "error out"=w1006:errorcluster)  [unwired: 13 in]
        n274 = Unbundle By Name(w970) -> ("V2 Step"=w971:dbl, "V2 Start"=w969:dbl, "Number of points"=w968:i32)
        n275 = Open/Create/Replace File(file path (use dialog)=w1010, error in=w1006, operation (0:open)=w962) -> (refnum out=w1020:refnum<file>, error out=w1021:errorcluster)  [unwired: 3 in, 1 out]
        n276 = call "4155C Make Big 2d array FPP.vi"("1D Var1"=w967, "1d ID"=w965, "1d Vp2"=w966, "1d IG"=w964, "1d Vp1"=w963, "VAR2 START"=w969, "Number of VAR2 steps"=w968, "VAR2 STEP"=w971, "VAR1 Name"="Vd", "Decimal places in header"=i8 1, "VAR2 Name"="Vg") -> ("Header array"=w1016:string[], "Data array"=w1017:dbl[][])  [unwired: 15 in]
        n277 = call "4155C Write array to file.vi"("Byte Stream File Refnum"=w1020, "Header"=w1016, "Data Array"=w1017, "error in (no error)"=w1021) -> ("dup refnum"=w1018:refnum<file>, "error out"=w1019:errorcluster)  [unwired: 1 in]
        n278 = Close File(refnum=w1018, error in=w1019) -> (error out=w1004:errorcluster)  [unwired: 1 out]
      }
      frame "itime" {
        n279 = Delete From Array(array=w1035, index=1) -> (deleted portion=w1034:string)  [unwired: 1 in, 1 out]
        n280 = Delete From Array(array=w1035, index=0 ("Index")) -> (deleted portion=w1063:string)  [unwired: 1 in, 1 out]
        n281 = Fract/Exp String To Number(string=w1034) -> (number=w1033:dbl)  [unwired: 3 in, 1 out]
        n282 = case shown="\"l\"" w1063 {
          tunnel: w1062 -> [w1068 w1070 w1074]
          tunnel: [w1067 w1069 w1073] -> w1055
          tunnel: w1033 -> [w1065 _ w1072]
          frame "s" {
            w1066 = u32 0 items=["short  ", "medium  ", "long  "] ("integration time 2")
            n283 = Bundle By Name(cluster=w1068, "integration time"=w1066, "Short/Long integration time"=w1065) -> (w1067:T4)
          }
          frame "m", Default {
            w1071 = u32 1 items=["short  ", "medium  ", "long  "] ("integration time 2")
            n284 = Bundle By Name(cluster=w1070, "integration time"=w1071) -> (w1069:T4)
          }
          frame "l" {
            w1075 = u32 2 items=["short  ", "medium  ", "long  "] ("integration time 2")
            n285 = Bundle By Name(cluster=w1074, "integration time"=w1075, "Short/Long integration time"=w1072) -> (w1073:T4)
          }
        }
      }
      frame "pulsed" {
        n286 = Delete From Array(array=w1108, index=0 ("Index")) -> (deleted portion=w1109:string, array with subset deleted=w1096:string[])  [unwired: 1 in]
        n287 = case shown="\"on\", Default" w1109 {
          tunnel: w1107 -> [w1119 w1122]
          tunnel: [w1118 w1121] -> w1100
          tunnel: w1096 -> [w1116 _]
          frame "on", Default {
            w1117 = u16 1 items=["Continuous", "Pulsed"] ("sweep method")
            n288 = Fract/Exp String To Number(string=w1116) -> (number=w1114:dbl[])  [unwired: 3 in, 1 out]
            n289 = Index Array(array=w1114, index #1=0 ("Index")) -> (element #1=w1113:dbl, element #2=w1112:dbl, element #3=w1111:dbl)  [unwired: 2 in]
            n290 = Bundle By Name(cluster=w1119, "sweep method"=w1117, "Pulse period"=w1113, "Base voltage"=w1112, "Pulse width"=w1111) -> (w1118:T4)
          }
          frame "off" {
            w1120 = u16 0 items=["Continuous", "Pulsed"] ("sweep method")
            n291 = Bundle By Name(cluster=w1122, "sweep method"=w1120) -> (w1121:T4)
          }
        }
      }
      frame "gaterangemode" {
        n292 = Delete From Array(array=w1153, index=0 ("Index")) -> (deleted portion=w1154:string)  [unwired: 1 in, 1 out]
        n293 = case shown="\"f\"" w1154 {
          tunnel: [w1156 w1157 w1158] -> w1143
          frame "a", Default {
            w1156 = u16 0 items=["Auto", "Limited", "Fixed"] ("Gate Range\nmode 2")
          }
          frame "f" {
            w1157 = u16 2 items=["Auto", "Limited", "Fixed"] ("Gate Range\nmode 2")
          }
          frame "l" {
            w1158 = u16 1 items=["Auto", "Limited", "Fixed"] ("Gate Range\nmode 2")
          }
        }
      }
      frame "gaterange" {
        (unwired) u8 11 items=["10fA  ", "100fA  ", "1nA  ", "10nA", "100nA", "1uA", "10uA", "100uA", "1mA", "10mA", "100mA", "1A"] ("Gate Range 2")
        n294 = Delete From Array(array=w1196, index=0 ("Index")) -> (deleted portion=w1186:string)  [unwired: 1 in, 1 out]
        n295 = Scan Value(string=w1186, format string="") -> (value=w1184:dbl)  [unwired: 1 in, 1 out]
        n296 = Logarithm Base 10(1:w1184) -> (0:w1183:dbl)
        n297 = Round To Nearest(number=w1183) -> (nearest integer value=w1182:dbl)
        n298 = Add(x=w1182, y=11.0) -> (x+y=w1180:dbl)
        n299 = To Unsigned Byte Integer(number=w1180) -> (unsigned 8bit integer=w1179:u8)
      }
      frame "drainrange" {
        (unwired) u8 11 items=["10fA  ", "100fA  ", "1nA  ", "10nA", "100nA", "1uA", "10uA", "100uA", "1mA", "10mA", "100mA", "1A"] ("Gate Range 2")
        n300 = Delete From Array(array=w1235, index=0 ("Index")) -> (deleted portion=w1226:string)  [unwired: 1 in, 1 out]
        n301 = Scan Value(string=w1226, format string="") -> (value=w1224:dbl)  [unwired: 1 in, 1 out]
        n302 = Logarithm Base 10(1:w1224) -> (0:w1223:dbl)
        n303 = Round To Nearest(number=w1223) -> (nearest integer value=w1222:dbl)
        n304 = Add(x=w1222, y=11.0) -> (x+y=w1220:dbl)
        n305 = To Unsigned Byte Integer(number=w1220) -> (unsigned 8bit integer=w1219:u8)
      }
      frame "drainrangemode" {
        n306 = Delete From Array(array=w1267, index=0 ("Index")) -> (deleted portion=w1268:string)  [unwired: 1 in, 1 out]
        n307 = case shown="\"f\"" w1268 {
          tunnel: [w1270 w1271 w1272] -> w1257
          frame "a", Default {
            w1270 = u16 0 items=["Auto", "Limited", "Fixed"] ("Gate Range\nmode 2")
          }
          frame "f" {
            w1271 = u16 2 items=["Auto", "Limited", "Fixed"] ("Gate Range\nmode 2")
          }
          frame "l" {
            w1272 = u16 1 items=["Auto", "Limited", "Fixed"] ("Gate Range\nmode 2")
          }
        }
      }
      frame "Error", Default {
      }
      frame "logfile" {
        n308 = Number To Decimal String(number=w1323) -> (decimal integer string=w1358:string)  [unwired: 1 in]
        n309 = Concatenate Strings(w1357, "logfile" ("Substring"), w1358, w1321, ".txt" ("Substring")) -> (w1355:string)
        n310 = String To Path(string=w1355) -> (path=w1328:path)
        n311 = Unbundle(w1354) -> ("integration time"=w1353:u32, "Short/Long integration time"=w1352:dbl, "hold time (sec)"=w1351:dbl, "delay time (sec)"=w1350:dbl, "Step Time (0 disables)"=w1349:dbl, "sweep method"=w1348:u16, "Pulse period"=w1347:dbl, "Base voltage"=w1346:dbl, "Pulse width"=w1345:dbl)
        n312 = Build Array(w1353, w1352, w1351, w1350, w1349, w1348, w1347, w1346, w1345, w1339, w1340, w1341, w1342, w1343, w1344) -> (w1332:dbl[])
        n313 = Insert Into Array(array=dbl[][] [] ("Input Array"), new element=w1332) -> (w1331:dbl[][])  [unwired: 2 in]
        n314 = call <vilib>:"compatOverwrite.vi"("overwrite (F)"=TRUE) -> ("overwrite?"=w1326:T8)
        n315 = Open/Create/Replace File(file path (use dialog)=w1328, error in=w1330, operation (0:open)=w1326) -> (refnum out=w1336:refnum<file>, error out=w1335:errorcluster)  [unwired: 3 in, 1 out]
        n316 = call "4155C Write array to file.vi"("Byte Stream File Refnum"=w1336, "Header"=string[] ["Int Time", "Short/Long Itime", "Hold time", "Delay time", "Step time", "Sweep method", "Pulse period", "Base Voltage", "Pulse width", "Drain compliance", "Gate compliance", "Gate range mode", "Gate range", "S/D range mode", "S/D range"], "Data Array"=w1331, "error in (no error)"=w1335) -> ("dup refnum"=w1338:refnum<file>, "error out"=w1337:errorcluster)  [unwired: 1 in]
        n317 = Close File(refnum=w1338, error in=w1337) -> (error out=w1329:errorcluster)  [unwired: 1 out]
      }
      frame "sample" {
        w1375 = 1
        # "Add a time offset (elapsed time) to the time axis."
        # "Adjusts graph colors."
        n318 = Number To Decimal String(number=w1407) -> (decimal integer string=w1449:string)  [unwired: 1 in]
        n319 = Fract/Exp String To Number(string=w1446) -> (number=w1411:dbl[])  [unwired: 3 in, 1 out]
        n320 = Concatenate Strings(w1427, "-sample-" ("Substring"), w1449, w1405, ".txt" ("Substring")) -> (w1447:string)
        n321 = Index Array(array=w1411, index=0 ("Index")) -> (element=w1444:dbl)
        n322 = String To Path(string=w1447) -> (path=w1431:path)
        n323 = Index Array(array=w1411, index=2 ("Index")) -> (element=w1440:dbl)
        n324 = Index Array(array=w1411, index=3 ("Index")) -> (element=w1413:dbl)
        n325 = Index Array(array=w1411, index=4 ("Index")) -> (element=w1410:dbl)
        n326 = call "4155C Config Sampling Measurements.vi"("Sampling interval"=w1410, "Sample time"=w1413, "Display on/off"=TRUE, "Timings"=w1419, "Num Points"=w1440, "error in (no error)"=w1451, "Drain Compliance"=w1450, "Gate Compliance"=w1428, "VISA session"=w1452) -> ("error out"=w1453:errorcluster, "dup VISA resource name"=w1454:refnum<visa-resource-name>)  [unwired: 1 in]
        n327 = Index Array(array=w1411, index=1 ("Index")) -> (element=w1441:dbl)
        n328 = local read "Plot sample extrema vs time"() -> (w1378:bool)
        n329 = call "4155C Take Sample.vi"("Emergency Stop"=w1424, "error in (no error)"=w1453, "Vd"=w1441, "Vg"=w1444, "VISA resource name in"=w1454) -> ("error out"=w1376:errorcluster, "Id"=w1370:dbl[], "Ig"=w1369:dbl[], "VISA Resource Name out"=w1421:refnum<visa-resource-name>, "Is"=w1371:dbl[], "Time"=w1374:dbl[])  [unwired: 1 in]
        n330 = Insert Into Array(array=w1367, new element=w1370) -> (w1361:dbl[])  [unwired: 1 in]
        n331 = Add(x=w1374, y=w1373) -> (x+y=w1372:dbl[])
        n332 = Insert Into Array(array=w1366, new element=w1371) -> (w1362:dbl[])  [unwired: 1 in]
        n333 = Insert Into Array(array=w1368, new element=w1369) -> (w1364:dbl[])  [unwired: 1 in]
        n334 = case shown="True" w1378 {
          tunnel: w1379 -> [w1455 w1457]
          tunnel: [w1455 w1458] -> w1377
          tunnel: w1372 -> [_ w1456]
          frame False {
          }
          frame True {
            n335 = Insert Into Array(array=w1457, new element=w1456) -> (w1458:i32[])  [unwired: 1 in]
          }
        }
        n336 = case shown="True" "Plot sample extrema vs time" {
          tunnel: w1371 -> [_ w1486]
          tunnel: w1370 -> [_ w1487]
          tunnel: w1369 -> [_ w1488]
          tunnel: [w1465 w1475] -> w1360
          tunnel: w1376 -> [w1465 w1479]
          tunnel: w1400 -> [w1464 w1491]
          tunnel: w1399 -> [w1463 w1490]
          tunnel: w1398 -> [w1462 w1492]
          tunnel: w1397 -> [w1461 w1489]
          tunnel: w1396 -> [w1460 w1494]
          tunnel: w1395 -> [w1459 w1493]
          tunnel: [w1464 w1477] -> w1394
          tunnel: [w1463 w1470] -> w1393
          tunnel: [w1462 w1471] -> w1392
          tunnel: [w1461 w1495] -> w1391
          tunnel: [w1460 w1478] -> w1390
          tunnel: [w1459 w1472] -> w1389
          tunnel: w1377 -> [_ w1466]
          frame False {
          }
          frame True {
            w1473 = 1
            # "Number of VAR2 steps is 1."
            # "abs(Ig)"
            # "abs(Is)"
            # "abs(Id)"
            # "Adjusts graph colors."
            n337 = Absolute Value(x=w1488) -> (abs(x)=w1467:dbl[])
            n338 = Absolute Value(x=w1487) -> (abs(x)=w1468:dbl[])
            n339 = Absolute Value(x=w1486) -> (abs(x)=w1469:dbl[])
            n340 = Array Max & Min(array=w1469) -> (max value=w1485:dbl, min value=w1482:dbl)  [unwired: 2 out]
            n341 = Array Max & Min(array=w1468) -> (max value=w1484:dbl, min value=w1481:dbl)  [unwired: 2 out]
            n342 = Array Max & Min(array=w1467) -> (max value=w1483:dbl, min value=w1480:dbl)  [unwired: 2 out]
            n343 = local write "Id max"(w1484) -> ()
            n344 = local write "Id min"(w1481) -> ()
            n345 = local write "Ig max"(w1483) -> ()
            n346 = local write "Ig min"(w1480) -> ()
            n347 = Insert Into Array(array=w1494, new element=w1467) -> (w1478:dbl[])  [unwired: 1 in]
            n348 = Insert Into Array(array=w1493, new element=w1467) -> (w1472:dbl[])  [unwired: 1 in]
            n349 = local write "Is max"(w1485) -> ()
            n350 = local write "Is min"(w1482) -> ()
            n351 = Insert Into Array(array=w1492, new element=w1468) -> (w1471:dbl[])  [unwired: 1 in]
            n352 = Insert Into Array(array=w1489, new element=w1468) -> (w1495:dbl[])  [unwired: 1 in]
            n353 = Insert Into Array(array=w1491, new element=w1469) -> (w1477:dbl[])  [unwired: 1 in]
            n354 = Insert Into Array(array=w1490, new element=w1469) -> (w1470:dbl[])  [unwired: 1 in]
            n355 = control-ref of="Imax vs time"() -> (w1496:refnum<vi>)
            n356 = call "4155C Config Chart Colours.vi"("Numeric"=w1473, "XY Graph 2"=w1496) -> ()  [unwired: 6 in]
            n357 = call "4155C Split array.vi"("Number of VAR2 steps"=w1473, "Y2 data in"=w1471, "X data in"=w1466, "Y1 data in"=w1477, "Y3 data in"=w1478, "error in (no error)"=w1479) -> ("Array of clusters"=w1497:cluster{"Y data in":dbl[], "X data in":dbl[]}[], "error out"=w1476:errorcluster)  [unwired: 1 in]
            n358 = call "4155C Split array.vi"("Number of VAR2 steps"=w1473, "Y2 data in"=w1471, "X data in"=w1466, "Y1 data in"=w1470, "Y3 data in"=w1472, "error in (no error)"=w1476) -> ("Array of clusters"=w1474:cluster{"Y data in":dbl[], "X data in":dbl[]}[], "error out"=w1475:errorcluster)  [unwired: 1 in]
            n359 = local write "Imax vs time"(w1497) -> ()
            n360 = local write "Imin vs time"(w1474) -> ()
          }
        }
        n361 = Insert Into Array(array=w1365, new element=w1372) -> (w1363:dbl[])  [unwired: 1 in]
        n362 = control-ref of="I vs time (Bias Stress)"() -> (w1382:refnum<vi>)
        n363 = call "4155C Split array.vi"("Number of VAR2 steps"=w1375, "Y2 data in"=w1361, "X data in"=w1363, "Y1 data in"=w1362, "Y3 data in"=w1364) -> ("Array of clusters"=w1381:cluster{"Y data in":dbl[], "X data in":dbl[]}[])  [unwired: 2 in, 1 out]
        n364 = call "4155C Config Chart Colours.vi"("Numeric"=w1375, "XY Graph 2"=w1382) -> ()  [unwired: 6 in]
        n365 = local write "I vs time (Bias Stress)"(w1381) -> ()
        n366 = Insert Into Array(array=dbl[][] [] ("Input Array"), new element=w1372) -> (w1380:dbl[][])  [unwired: 2 in]
        n367 = Insert Into Array(array=w1380, new element=w1369) -> (w1434:dbl[][])  [unwired: 2 in]
        n368 = VISA Write(VISA resource name=w1421, write buffer=":DISP ON" ("write buffer (\"\")"), error in (no error)=w1360) -> (VISA resource name out=w1420:refnum<visa-resource-name>, error out=w1422:errorcluster)  [unwired: 1 out]
        n369 = Insert Into Array(array=w1434, new element=w1370) -> (w1433:dbl[][])  [unwired: 2 in]
        n370 = Insert Into Array(array=w1433, new element=w1371) -> (w1426:dbl[][])  [unwired: 2 in]
        n371 = Transpose 2D Array(2D array=w1426) -> (transposed array=w1425:dbl[][])
        n372 = call <vilib>:"compatOverwrite.vi"("overwrite (F)"=TRUE) -> ("overwrite?"=w1408:T8)
        n373 = Open/Create/Replace File(file path (use dialog)=w1431, error in=w1422, operation (0:open)=w1408) -> (refnum out=w1437:refnum<file>, error out=w1436:errorcluster)  [unwired: 3 in, 1 out]
        n374 = call "4155C Write array to file.vi"("Byte Stream File Refnum"=w1437, "Header"=string[] ["Time /s", "Ig /A", "Id /A", "Is /A"], "Data Array"=w1425, "error in (no error)"=w1436) -> ("dup refnum"=w1439:refnum<file>, "error out"=w1438:errorcluster)  [unwired: 1 in]
        n375 = Close File(refnum=w1439, error in=w1438) -> (error out=w1429:errorcluster)  [unwired: 1 out]
      }
      frame "samplei" {
        n376 = Number To Decimal String(number=w1518) -> (decimal integer string=w1569:string)  [unwired: 1 in]
        n377 = Concatenate Strings(w1548, "-samplei-" ("Substring"), w1569, w1517, ".txt" ("Substring")) -> (w1567:string)
        n378 = Fract/Exp String To Number(string=w1566) -> (number=w1533:dbl[])  [unwired: 3 in, 1 out]
        n379 = String To Path(string=w1567) -> (path=w1551:path)
        n380 = Index Array(array=w1533, index=4 ("Index")) -> (element=w1527:dbl)
        n381 = Index Array(array=w1533, index=3 ("Index")) -> (element=w1528:dbl)
        n382 = Index Array(array=w1533, index=1 ("Index")) -> (element=w1530:dbl)
        n383 = Index Array(array=w1533, index=0 ("Index")) -> (element=w1531:dbl)
        n384 = Index Array(array=w1533, index=2 ("Index")) -> (element=w1529:dbl)
        n385 = call "4155C Config SamplingI Measurements.vi"("Sample time"=w1529, "Display on/off"=TRUE, "Timings"=w1540, "Num Points"=w1530, "error in (no error)"=w1571, "Sampling interval"=w1528, "VISA session"=w1572) -> ("error out"=w1573:errorcluster, "dup VISA resource name"=w1574:refnum<visa-resource-name>)  [unwired: 3 in]
        n386 = call "4155C Take SampleI.vi"("Emergency Stop"=w1545, "error in (no error)"=w1573, "Idg 2"=w1531, "Vdg compliance 2"=w1527, "VISA resource name in"=w1574) -> ("error out"=w1543:errorcluster, "Idg"=w1576:dbl[], "Vdg"=w1553:dbl[], "VISA Resource Name out"=w1541:refnum<visa-resource-name>, "Is"=w1575:dbl[], "Time"=w1557:dbl[])  [unwired: 1 in]
        n387 = Insert Into Array(array=dbl[][] [] ("Input Array"), new element=w1557) -> (w1556:dbl[][])  [unwired: 2 in]
        n388 = Insert Into Array(array=w1556, new element=w1553) -> (w1555:dbl[][])  [unwired: 2 in]
        n389 = Insert Into Array(array=w1555, new element=w1576) -> (w1554:dbl[][])  [unwired: 2 in]
        n390 = VISA Write(VISA resource name=w1541, write buffer=":DISP ON" ("write buffer (\"\")"), error in (no error)=w1543) -> (VISA resource name out=w1526:refnum<visa-resource-name>, error out=w1542:errorcluster)  [unwired: 1 out]
        n391 = Insert Into Array(array=w1554, new element=w1575) -> (w1547:dbl[][])  [unwired: 2 in]
        n392 = call <vilib>:"compatOverwrite.vi"("overwrite (F)"=TRUE) -> ("overwrite?"=w1521:T8)
        n393 = Open/Create/Replace File(file path (use dialog)=w1551, error in=w1542, operation (0:open)=w1521) -> (refnum out=w1560:refnum<file>, error out=w1559:errorcluster)  [unwired: 3 in, 1 out]
        n394 = Transpose 2D Array(2D array=w1547) -> (transposed array=w1546:dbl[][])
        n395 = call "4155C Write array to file.vi"("Byte Stream File Refnum"=w1560, "Header"=string[] ["Time /s", "Vdg /V", "Idg /A", "Is /A"], "Data Array"=w1546, "error in (no error)"=w1559) -> ("dup refnum"=w1562:refnum<file>, "error out"=w1561:errorcluster)  [unwired: 1 in]
        n396 = Close File(refnum=w1562, error in=w1561) -> (error out=w1524:errorcluster)  [unwired: 1 out]
        n397 = VISA Write(VISA resource name=w1526, write buffer=";:PAGE:SCON:STAN OFF;:PAGE:CHAN:VSU2:DIS;" ("write buffer (\"\")"), error in (no error)=w1524) -> (VISA resource name out=w1522:refnum<visa-resource-name>, error out=w1523:errorcluster)  [unwired: 1 out]
      }
      frame "#" {
        n398 = VISA Write(VISA resource name=w1601, write buffer=":DISP ON" ("write buffer (\"\")"), error in (no error)=w1600) -> (VISA resource name out=w1599:refnum<visa-resource-name>, error out=w1598:errorcluster)  [unwired: 1 out]
      }
      frame "stressV" {
        n399 = Number To Decimal String(number=w1629) -> (decimal integer string=w1670:string)  [unwired: 1 in]
        n400 = Concatenate Strings(w1654, "-stressV-" ("Substring"), w1670, w1628, ".txt" ("Substring")) -> (w1668:string)
        n401 = Fract/Exp String To Number(string=w1667) -> (number=w1640:dbl[])  [unwired: 3 in, 1 out]
        n402 = String To Path(string=w1668) -> (path=w1658:path)
        n403 = Index Array(array=w1640, index=3 ("Index")) -> (element=w1637:dbl)
        n404 = Index Array(array=w1640, index=1 ("Index")) -> (element=w1635:dbl)
        n405 = Index Array(array=w1640, index=0 ("Index")) -> (element=w1634:dbl)
        n406 = Index Array(array=w1640, index=4 ("Index")) -> (element=w1639:dbl)
        n407 = Index Array(array=w1640, index=2 ("Index")) -> (element=w1636:dbl)
        n408 = call "4155C Config V Stress.vi"("VISA session"=w1673, "ID compliance"=w1637, "VD"=w1635, "VG"=w1634, "IG compliance"=w1636, "error in (no error)"=w1672, "Display on/off"=TRUE) -> ("dup VISA resource name"=w1675:refnum<visa-resource-name>, "error out"=w1674:errorcluster)
        n409 = call "4155C Apply Stress.vi"("error in (no error)"=w1674, "Duration"=w1639, "Emergency Stop"=w1653, "VISA resource name in"=w1675) -> ("error out"=w1651:errorcluster, "VISA Resource Name out"=w1649:refnum<visa-resource-name>)
        n410 = VISA Write(VISA resource name=w1649, write buffer=":DISP ON" ("write buffer (\"\")"), error in (no error)=w1651) -> (VISA resource name out=w1648:refnum<visa-resource-name>, error out=w1650:errorcluster)  [unwired: 1 out]
        n411 = call <vilib>:"compatOverwrite.vi"("overwrite (F)"=TRUE) -> ("overwrite?"=w1633:T8)
        n412 = Open/Create/Replace File(file path (use dialog)=w1658, error in=w1650, operation (0:open)=w1633) -> (refnum out=w1661:refnum<file>, error out=w1660:errorcluster)  [unwired: 3 in, 1 out]
        n413 = call "4155C Write array to file.vi"("Byte Stream File Refnum"=w1661, "Header"=string[] ["V stress completed successfully", ""], "error in (no error)"=w1660) -> ("dup refnum"=w1663:refnum<file>, "error out"=w1662:errorcluster)  [unwired: 2 in]
        n414 = Close File(refnum=w1663, error in=w1662) -> (error out=w1656:errorcluster)  [unwired: 1 out]
      }
      frame "stressI" {
        n415 = Number To Decimal String(number=w1695) -> (decimal integer string=w1732:string)  [unwired: 1 in]
        n416 = Concatenate Strings(w1716, "-stressI-" ("Substring"), w1732, w1694, ".txt" ("Substring")) -> (w1730:string)
        n417 = Fract/Exp String To Number(string=w1729) -> (number=w1704:dbl[])  [unwired: 3 in, 1 out]
        n418 = Index Array(array=w1704, index=1 ("Index")) -> (element=w1700:dbl)
        n419 = Index Array(array=w1704, index=0 ("Index")) -> (element=w1701:dbl)
        n420 = call "4155C Config I Stress.vi"("VISA session"=w1735, "IDG"=w1701, "VDG compliance"=w1700, "error in (no error)"=w1734, "Display on/off"=TRUE) -> ("dup VISA resource name"=w1737:refnum<visa-resource-name>, "error out"=w1736:errorcluster)
        n421 = Index Array(array=w1704, index=2 ("Index")) -> (element=w1702:dbl)
        n422 = String To Path(string=w1730) -> (path=w1720:path)
        n423 = call "4155C Apply Stress.vi"("error in (no error)"=w1736, "Duration"=w1702, "Emergency Stop"=w1715, "VISA resource name in"=w1737) -> ("error out"=w1713:errorcluster, "VISA Resource Name out"=w1711:refnum<visa-resource-name>)
        n424 = VISA Write(VISA resource name=w1711, write buffer=":DISP ON" ("write buffer (\"\")"), error in (no error)=w1713) -> (VISA resource name out=w1710:refnum<visa-resource-name>, error out=w1712:errorcluster)  [unwired: 1 out]
        n425 = call <vilib>:"compatOverwrite.vi"("overwrite (F)"=TRUE) -> ("overwrite?"=w1699:T8)
        n426 = Open/Create/Replace File(file path (use dialog)=w1720, error in=w1712, operation (0:open)=w1699) -> (refnum out=w1723:refnum<file>, error out=w1722:errorcluster)  [unwired: 3 in, 1 out]
        n427 = call "4155C Write array to file.vi"("Byte Stream File Refnum"=w1723, "Header"=string[] ["I stress completed successfully", ""], "error in (no error)"=w1722) -> ("dup refnum"=w1725:refnum<file>, "error out"=w1724:errorcluster)  [unwired: 2 in]
        n428 = Close File(refnum=w1725, error in=w1724) -> (error out=w1718:errorcluster)  [unwired: 1 out]
      }
      frame "vsu2pulse" {
        n429 = Number To Decimal String(number=w1757) -> (decimal integer string=w1792:string)  [unwired: 1 in]
        n430 = Concatenate Strings(w1777, "-vsu2-" ("Substring"), w1792, w1756, ".txt" ("Substring")) -> (w1790:string)
        n431 = Fract/Exp String To Number(string=w1789) -> (number=w1765:dbl[])  [unwired: 3 in, 1 out]
        n432 = String To Path(string=w1790) -> (path=w1781:path)
        n433 = Index Array(array=w1765, index=1 ("Index")) -> (element=w1764:dbl)
        n434 = Index Array(array=w1765, index=0 ("Index")) -> (element=w1762:dbl)
        n435 = call "4155C Config VSU2 Stress.vi"("error in (no error)"=w1794, "VSU2"=w1762, "Display on/off"=TRUE, "VISA session"=w1795) -> ("error out"=w1796:errorcluster, "dup VISA resource name"=w1797:refnum<visa-resource-name>)
        n436 = call "4155C Apply Stress.vi"("error in (no error)"=w1796, "Duration"=w1764, "Emergency Stop"=w1776, "VISA resource name in"=w1797) -> ("error out"=w1774:errorcluster, "VISA Resource Name out"=w1772:refnum<visa-resource-name>)
        n437 = VISA Write(VISA resource name=w1772, write buffer=":DISP ON" ("write buffer (\"\")"), error in (no error)=w1774) -> (VISA resource name out=w1771:refnum<visa-resource-name>, error out=w1773:errorcluster)  [unwired: 1 out]
        n438 = call <vilib>:"compatOverwrite.vi"("overwrite (F)"=TRUE) -> ("overwrite?"=w1761:T8)
        n439 = Open/Create/Replace File(file path (use dialog)=w1781, error in=w1773, operation (0:open)=w1761) -> (refnum out=w1784:refnum<file>, error out=w1783:errorcluster)  [unwired: 3 in, 1 out]
        n440 = call "4155C Write array to file.vi"("Byte Stream File Refnum"=w1784, "Header"=string[] ["VSU2 pulse completed successfully", ""], "error in (no error)"=w1783) -> ("dup refnum"=w1786:refnum<file>, "error out"=w1785:errorcluster)  [unwired: 2 in]
        n441 = Close File(refnum=w1786, error in=w1785) -> (error out=w1779:errorcluster)  [unwired: 1 out]
      }
      frame "sample-fpp" {
        w1828 = string[] ["Time /s", "Id VgVd /A", "Ig VgVd /A", "Vp1 VgVd /V", "Vp2 VgVd /V"] ("Header")
        w1832 = "%d" ("format string")
        n442 = Number To Decimal String(number=w1817) -> (decimal integer string=w1880:string)  [unwired: 1 in]
        n443 = Fract/Exp String To Number(string=w1877) -> (number=w1865:dbl[])  [unwired: 3 in, 1 out]
        n444 = Concatenate Strings(w1871, "-samplefpp-" ("Substring"), w1880, w1816, ".txt" ("Substring")) -> (w1878:string)
        n445 = String To Path(string=w1878) -> (path=w1840:path)
        n446 = Index Array(array=w1865, index=0 ("Index")) -> (element=w1826:dbl)
        n447 = Index Array(array=w1865, index=1 ("Index")) -> (element=w1825:dbl)
        n448 = Index Array(array=w1865, index=2 ("Index")) -> (element=w1873:dbl)
        n449 = Index Array(array=w1865, index=3 ("Index")) -> (element=w1863:dbl)
        n450 = call "4155C Config Sampling Measurements FPP.vi"("VISA session"=w1883, "Num Points"=w1873, "Vg"=w1826, "Display on/off"=TRUE, "Gate Compliance"=w1872, "Drain Compliance"=w1881, "Standby"="Standby", "error in (no error)"=w1882, "Timings"=w1870, "Vd"=w1825, "Sample time"=w1863) -> ("dup VISA resource name"=w1842:refnum<visa-resource-name>, "error out"=w1841:errorcluster)  [unwired: 3 in]
        n451 = Number To Decimal String(number=w1826) -> (decimal integer string=w1852:string)  [unwired: 1 in]
        n452 = call "4155C Take Sample FPP.vi"("VISA resource name in"=w1842, "error in (no error)"=w1841, "Emergency Stop"=w1843) -> ("Time"=w1847:dbl[], "Vp1"=w1857:dbl[], "VISA Resource Name out"=w1823:refnum<visa-resource-name>, "Ig"=w1845:dbl[], "Id"=w1846:dbl[], "Vp2"=w1855:dbl[], "error out"=w1844:errorcluster)  [unwired: 10 in]
        n453 = Insert Into Array(array=dbl[][] [] ("Input Array"), new element=w1847) -> (w1861:dbl[][])  [unwired: 2 in]
        n454 = Number To Decimal String(number=w1825) -> (decimal integer string=w1850:string)  [unwired: 1 in]
        n455 = Insert Into Array(array=w1861, new element=w1846) -> (w1860:dbl[][])  [unwired: 2 in]
        n456 = Concatenate Strings("(Vg = " ("Substring"), w1852, "V, Vd = " ("Substring"), w1850, "V)" ("Substring")) -> (w1848:string)
        n457 = Insert Into Array(array=w1860, new element=w1845) -> (w1859:dbl[][])  [unwired: 2 in]
        n458 = Insert Into Array(array=w1859, new element=w1857) -> (w1856:dbl[][])  [unwired: 2 in]
        n459 = Insert Into Array(array=w1856, new element=w1855) -> (w1824:dbl[][])  [unwired: 2 in]
        n460 = Transpose 2D Array(2D array=w1824) -> (transposed array=w1854:dbl[][])
        n461 = call <vilib>:"compatOverwrite.vi"("overwrite (F)"=TRUE) -> ("overwrite?"=w1821:T8)
        n462 = Open/Create/Replace File(file path (use dialog)=w1840, error in=w1844, operation (0:open)=w1821) -> (refnum out=w1837:refnum<file>, error out=w1838:errorcluster)  [unwired: 3 in, 1 out]
        n463 = Array To Spreadsheet String(array=w1828, 3:w1832) -> (spreadsheet string=w1834:string)  [unwired: 1 in]
        n464 = Search and Replace String(replace all?=TRUE ("replace all? (F)"), input string=w1834, search string="VgVd", replace string=w1848) -> (result string=w1830:string)  [unwired: 4 in, 3 out]
        n465 = Spreadsheet String To Array(format string=w1832, spreadsheet string=w1830, array type (2D Dbl)=w1828) -> (array=w1829:string[])  [unwired: 1 in]
        n466 = call "4155C Write array to file.vi"("Byte Stream File Refnum"=w1837, "Header"=w1829, "Data Array"=w1854, "error in (no error)"=w1838) -> ("dup refnum"=w1835:refnum<file>, "error out"=w1836:errorcluster)  [unwired: 1 in]
        n467 = Close File(refnum=w1835, error in=w1836) -> (error out=w1822:errorcluster)  [unwired: 1 out]
      }
      frame "resample-fpp" {
        w1916 = string[] ["Time /s", "Id VgVd /A", "Ig VgVd /A", "Vp1 VgVd /V", "Vp2 VgVd /V"] ("Header")
        w1920 = "%d" ("format string")
        n468 = Number To Decimal String(number=w1902) -> (decimal integer string=w1960:string)  [unwired: 1 in]
        n469 = Fract/Exp String To Number(string=w1957) -> (number=w1909:dbl[])  [unwired: 3 in, 1 out]
        n470 = Concatenate Strings(w1953, "-resamplefpp-" ("Substring"), w1960, w1903, ".txt" ("Substring")) -> (w1958:string)
        n471 = String To Path(string=w1958) -> (path=w1928:path)
        n472 = Index Array(array=w1909, index=0 ("Index")) -> (element=w1915:dbl)
        n473 = Index Array(array=w1909, index=1 ("Index")) -> (element=w1914:dbl)
        n474 = Number To Decimal String(number=w1915) -> (decimal integer string=w1938:string)  [unwired: 1 in]
        n475 = call "4155C Take Sample FPP.vi"("VISA resource name in"=w1911, "error in (no error)"=w1910, "Emergency Stop"=w1929) -> ("Time"=w1933:dbl[], "Vp1"=w1943:dbl[], "VISA Resource Name out"=w1913:refnum<visa-resource-name>, "Ig"=w1931:dbl[], "Id"=w1932:dbl[], "Vp2"=w1941:dbl[], "error out"=w1930:errorcluster)  [unwired: 10 in]
        n476 = Insert Into Array(array=dbl[][] [] ("Input Array"), new element=w1933) -> (w1947:dbl[][])  [unwired: 2 in]
        n477 = Number To Decimal String(number=w1914) -> (decimal integer string=w1936:string)  [unwired: 1 in]
        n478 = Insert Into Array(array=w1947, new element=w1932) -> (w1946:dbl[][])  [unwired: 2 in]
        n479 = Concatenate Strings("(Vg = " ("Substring"), w1938, "V, Vd = " ("Substring"), w1936, "V)" ("Substring")) -> (w1934:string)
        n480 = Insert Into Array(array=w1946, new element=w1931) -> (w1945:dbl[][])  [unwired: 2 in]
        n481 = Insert Into Array(array=w1945, new element=w1943) -> (w1942:dbl[][])  [unwired: 2 in]
        n482 = Insert Into Array(array=w1942, new element=w1941) -> (w1908:dbl[][])  [unwired: 2 in]
        n483 = call <vilib>:"compatOverwrite.vi"("overwrite (F)"=TRUE) -> ("overwrite?"=w1907:T8)
        n484 = Open/Create/Replace File(file path (use dialog)=w1928, error in=w1930, operation (0:open)=w1907) -> (refnum out=w1925:refnum<file>, error out=w1926:errorcluster)  [unwired: 3 in, 1 out]
        n485 = Array To Spreadsheet String(array=w1916, 3:w1920) -> (spreadsheet string=w1922:string)  [unwired: 1 in]
        n486 = Transpose 2D Array(2D array=w1908) -> (transposed array=w1940:dbl[][])
        n487 = Search and Replace String(replace all?=TRUE ("replace all? (F)"), input string=w1922, search string="VgVd", replace string=w1934) -> (result string=w1918:string)  [unwired: 4 in, 3 out]
        n488 = Spreadsheet String To Array(format string=w1920, spreadsheet string=w1918, array type (2D Dbl)=w1916) -> (array=w1917:string[])  [unwired: 1 in]
        n489 = call "4155C Write array to file.vi"("Byte Stream File Refnum"=w1925, "Header"=w1917, "Data Array"=w1940, "error in (no error)"=w1926) -> ("dup refnum"=w1923:refnum<file>, "error out"=w1924:errorcluster)  [unwired: 1 in]
        n490 = Close File(refnum=w1923, error in=w1924) -> (error out=w1912:errorcluster)  [unwired: 1 out]
      }
      frame "serial" {
        n491 = local read "Termination char\n(0xA = '\\n' = LF)\n(0xD = '\\r' = CR)"() -> (w1987:u8)
        n492 = local read "Enable Termination\nChar (T)"() -> (w1988:bool)
        n493 = Index Array(array=w1995, index=0 ("Index")) -> (element=w1994:string)
        n494 = local read "parity"() -> (w1978:u16)
        n495 = local read "Delay before read (ms)"() -> (w1989:u32)
        n496 = local read "byte count"() -> (w1986:u32)
        n497 = local read "Timeout (ms)"() -> (w1985:u32)
        n498 = local read "VISA resource name"() -> (w1982:refnum<visa-resource-name>)
        n499 = local read "baud rate"() -> (w1981:u32)
        n500 = local read "Serial End Mode for Reads"() -> (w1980:u16)
        n501 = local read "data bits"() -> (w1979:u16)
        n502 = local read "stop bits"() -> (w1984:u16)
        n503 = local read "flow control"() -> (w1983:u16)
        n504 = call "Serial write and read v0.5.vi"("Delay before read (ms)"=w1989, "Termination char\n(0xA = '\\n' = LF)\n(0xD = '\\r' = CR)"=w1987, "Enable Termination\nChar (T)"=w1988, "parity"=w1978, "stop bits"=w1984, "string to write"=w1994, "flow control"=w1983, "byte count"=w1986, "Serial Settings:Serial End Mode for Reads"=w1980, "Timeout (ms)"=w1985, "error in (no error)"=w2000, "VISA resource name"=w1982, "baud rate"=w1981, "data bits"=w1979) -> ("Serial port output"=w1990:string, "error out"=w1999:errorcluster)
        n505 = Build Array (concatenate)(w1990, w1991) -> (w1992:string[])
      }
    }
    n506 = local read "Time Units"() -> (w96:u16)
    n507 = case shown="0" w96 {
      tunnel: ["Time (Seconds)" ("element") "Time (Minutes)" ("element") "Time (Hours)" ("element")] -> w134
      frame 0 {
      }
      frame 1, Default {
      }
      frame 2 {
      }
    }
    n508 = Build Array(w146, w102, w112, w111, w110, w109, w108, w107, w106, w105, w104, w103, w101) -> (w167:dbl[][])
    n509 = Transpose 2D Array(2D array=w167) -> (transposed array=w166:dbl[][])
    n510 = Concatenate Strings(w68, "-Imax_Imin_Ion_Ioff_vs_time.txt" ("Suffix (Imax,Imin,Ion,Ioff)")) -> (w177:string)
    n511 = Build Array(w134, "Is max (A)" ("VAR2 Name"), "Is min (A)" ("VAR2 Name"), "Id max (A)" ("VAR2 Name"), "Id min (A)" ("VAR2 Name"), "Ig max (A)" ("VAR2 Name"), "Ig min (A)" ("VAR2 Name"), "Is on (A)" ("VAR2 Name"), "Is off (A)" ("VAR2 Name"), "Id on (A)" ("VAR2 Name"), "Id off (A)" ("VAR2 Name"), "Ig on (A)" ("VAR2 Name"), "Ig off (A)" ("VAR2 Name")) -> (w172:string[])
    n512 = Array To Spreadsheet String(array=w166, 3:"%e" ("format string")) -> (spreadsheet string=w170:string)  [unwired: 1 in]
    n513 = Array To Spreadsheet String(array=w172, 3:"" ("format string")) -> (spreadsheet string=w171:string)  [unwired: 1 in]
    n514 = String To Path(string=w177) -> (path=w176:path)
    n515 = Build Array(w171, w170) -> (w169:string[])
    n516 = Write to Text File(file (use dialog)=w176, text=w169, error in=w145) -> (refnum out=w178:refnum<file>, error out=w168:errorcluster)  [unwired: 1 in, 1 out]
    n517 = Close File(refnum=w178, error in=w168) -> (error out=w99:errorcluster)  [unwired: 1 out]
    n518 = Concatenate Strings(w68, "-serial_port_output.txt" ("Suffix (serial port log)")) -> (w148:string)
    n519 = String To Path(string=w148) -> (path=w147:path)
    n520 = Build Array(w134, "Serial port input" ("VAR2 Name"), "Serial port output: ") -> (w138:string[])
    n521 = Array To Spreadsheet String(array=w142, 3:"" ("format string")) -> (spreadsheet string=w135:string)  [unwired: 1 in]
    n522 = Array To Spreadsheet String(array=w138, 3:"" ("format string")) -> (spreadsheet string=w136:string)  [unwired: 1 in]
    n523 = Build Array(w136, w135) -> (w137:string[])
    n524 = Array To Spreadsheet String(array=w141, 3:"" ("format string")) -> (spreadsheet string=w153:string)  [unwired: 1 in]
    n525 = Write to Text File(file (use dialog)=w147, text=w137, error in=w99) -> (refnum out=w149:refnum<file>, error out=w150:errorcluster)  [unwired: 1 in, 1 out]
    n526 = Close File(refnum=w149, error in=w150) -> (error out=w70:errorcluster)  [unwired: 1 out]
    n527 = local write "Serial port data"(w153) -> ()
    n528 = Build Array(w67, w66, w65, w64) -> (w80:dbl[][])
    n529 = Build Array("Time (Seconds)" ("element"), "Is (A)" ("VAR2 Name"), "Id (A)" ("VAR2 Name"), "Ig (A)" ("VAR2 Name")) -> (w76:string[])
    n530 = Transpose 2D Array(2D array=w80) -> (transposed array=w79:dbl[][])
    n531 = Concatenate Strings(w68, "-sample_vs_time.txt" ("Suffix (Imax,Imin,Ion,Ioff)")) -> (w86:string)
    n532 = Array To Spreadsheet String(array=w76, 3:"" ("format string")) -> (spreadsheet string=w75:string)  [unwired: 1 in]
    n533 = Array To Spreadsheet String(array=w79, 3:"%e" ("format string")) -> (spreadsheet string=w83:string)  [unwired: 1 in]
    n534 = String To Path(string=w86) -> (path=w85:path)
    n535 = Build Array(w75, w83) -> (w82:string[])
    n536 = Write to Text File(file (use dialog)=w85, text=w82, error in=w70) -> (refnum out=w87:refnum<file>, error out=w81:errorcluster)  [unwired: 1 in, 1 out]
    n537 = Close File(refnum=w87, error in=w81) -> (error out=w69:errorcluster)  [unwired: 1 out]
  }
  "error out" <- w27
  "Timings Indicator" <- w19
  "SMU4 Indicator" <- w3
  "Is max" <- w13
  "Id max" <- w13
  "Ig max" <- w13
  "Imax vs time" <- w2
  "I vs Vg" <- w2
  "Imin vs time" <- w2
  "I vs Vd" <- w2
  "Serial port data" <- "" ("Serial port data")
  "Is min" <- w12
  "Id min" <- w12
  "Ig min" <- w12
  "Ion vs time" <- w2
  "Ioff vs time" <- w2
  "Is on" <- w11
  "Id on" <- w11
  "Ig on" <- w11
  "Is off" <- w10
  "Id off" <- w10
  "Ig off" <- w10
  "I vs time (Bias Stress)" <- w2
